vi "Auto_New.vi"() -> ()   [LabVIEW 2017]
uses:
  Control/Saurabh/prosucer_consumer_enum1.ctl
  <vilib>/Utility/error.llb/DialogType.ctl
  <vilib>/addons/database/Connection.llb/DB Tools Open Connec (String).vi
  Global/DATA LOG.vi
  Global/Global 1.vi
  <vilib>/addons/database/NI_Database_API.lvlib
panel:
  out "SHIFT":string
  in  "BARCODE RECIPE":string(combo)
  out "PLC COM.":bool
  out "SHIFT_DATA":string[](array[string])
  out "stop":bool
  out "error out 2":errorcluster
  out "Shift 4":i32
  out "Time Stamp Out":timestamp[](array[timestamp]) format="%<%X>T"
  out "Time Stamp Out 4":timestamp[](array[timestamp]) format="%<%X>T"
  out "Shift_change":bool
  out "appended array":string[][](array[string])
  out "SHIFT_DATA 2":string[](array[string])
  in  "error in (no error)":errorcluster
  in  "Tab Control":enum32{"Screen 1", "Screen 2"}(tab)
  out "OP 50":bool
  out "OP 40":bool
  out "OP 30":bool
  out "OP - 50":T1 {"RH Motor Screw" format="%#_g N-m"; "LH Motor Screw" format="%#_g N-m"; "Nut Torque" format="%#_g N-m"}
  out "OP - 40":T2 {"Stack Load" format="%#_g kg"; "Dispalcement" format="%#.3g mm"; "LH Screw" format="%#_g N-m"; "RH Screw" format="%#_g N-m"}
  out "OP - 30":T3 {"Shaft Press Load" format="%#_g kg"; "Displacement" format="%#_g mm"}
  in  "stop 2":bool
  out "OP - 10":T4 {"Leak Rate" format="%#_g sccm"}
  in  "SIMULATE INPUT":bool[](array[boolean])=[FALSE, FALSE, FALSE, FALSE]
  out "OP - 20":T5 {"Top Load" format="%#_g mm"; "Top Displace" format="%#_g mm"; "Bottom Load" format="%#_g kg"; "Bottom Displace" format="%#_g mm"}
  out "OP 10 & 20":bool
  out "OP - 60":T6 {"Screw 6" format="%#_g N-m"; "Screw 5" format="%#_g N-m"; "Screw 4" format="%#_g N-m"; "Screw 3" format="%#_g N-m"; "Screw 2" format="%#_g N-m"; "Screw 1" format="%#_g N-m"}
  out "OP - 70":T7 {"Full Open" format="%#_g V"; "Full Close" format="%#_g V"}
  out "OP - 110":cluster{"BARCODE":string}
  out "OP - 80":T8 {"Plug Press Load" format="%#_g kg"}
  out "OP - 90":T9 {"Steam Leak" format="%#_g sccm"; "Seat Leak" format="%#_g LPM"}
  out "OP - 100":T10 {"Response Time REV" format="%#_g msec"; "Response time FWD" format="%#_g msec"; "Motor Full Open" format="%#_g V"; "Motor Start Back" format="%#_g V"; "Motor Full Close" format="%#_g V"; "Motor Start Of Close" format="%#_g V"; "Motor Peak" format="%#_g A"; "Sensor O/P Full Close" format="%#_g V"; "Sensor O/P Start Of Close" format="%#_g V"; "Sensor O/P Open" format="%#_g V"}
  out "OP 60":bool
  out "OP 70 & 80":bool
  out "OP 90 -100 - 110":bool
  # "Op10 20\nOp30\nOp 40\nOp50\nOp60\nOp70-80\nOp 90-100-110"
  # "SENSOR MIN VLTG"
  # "OP - 50"
  # "OP - 40"
  # "OP - 30"
  # "OP - 10"
  # "OP - 20"
  # "OP - 60"
  # "OP - 70"
  # "OP - 110"
  # "OP - 80"
  # "OP - 90"
  # "OP - 100"
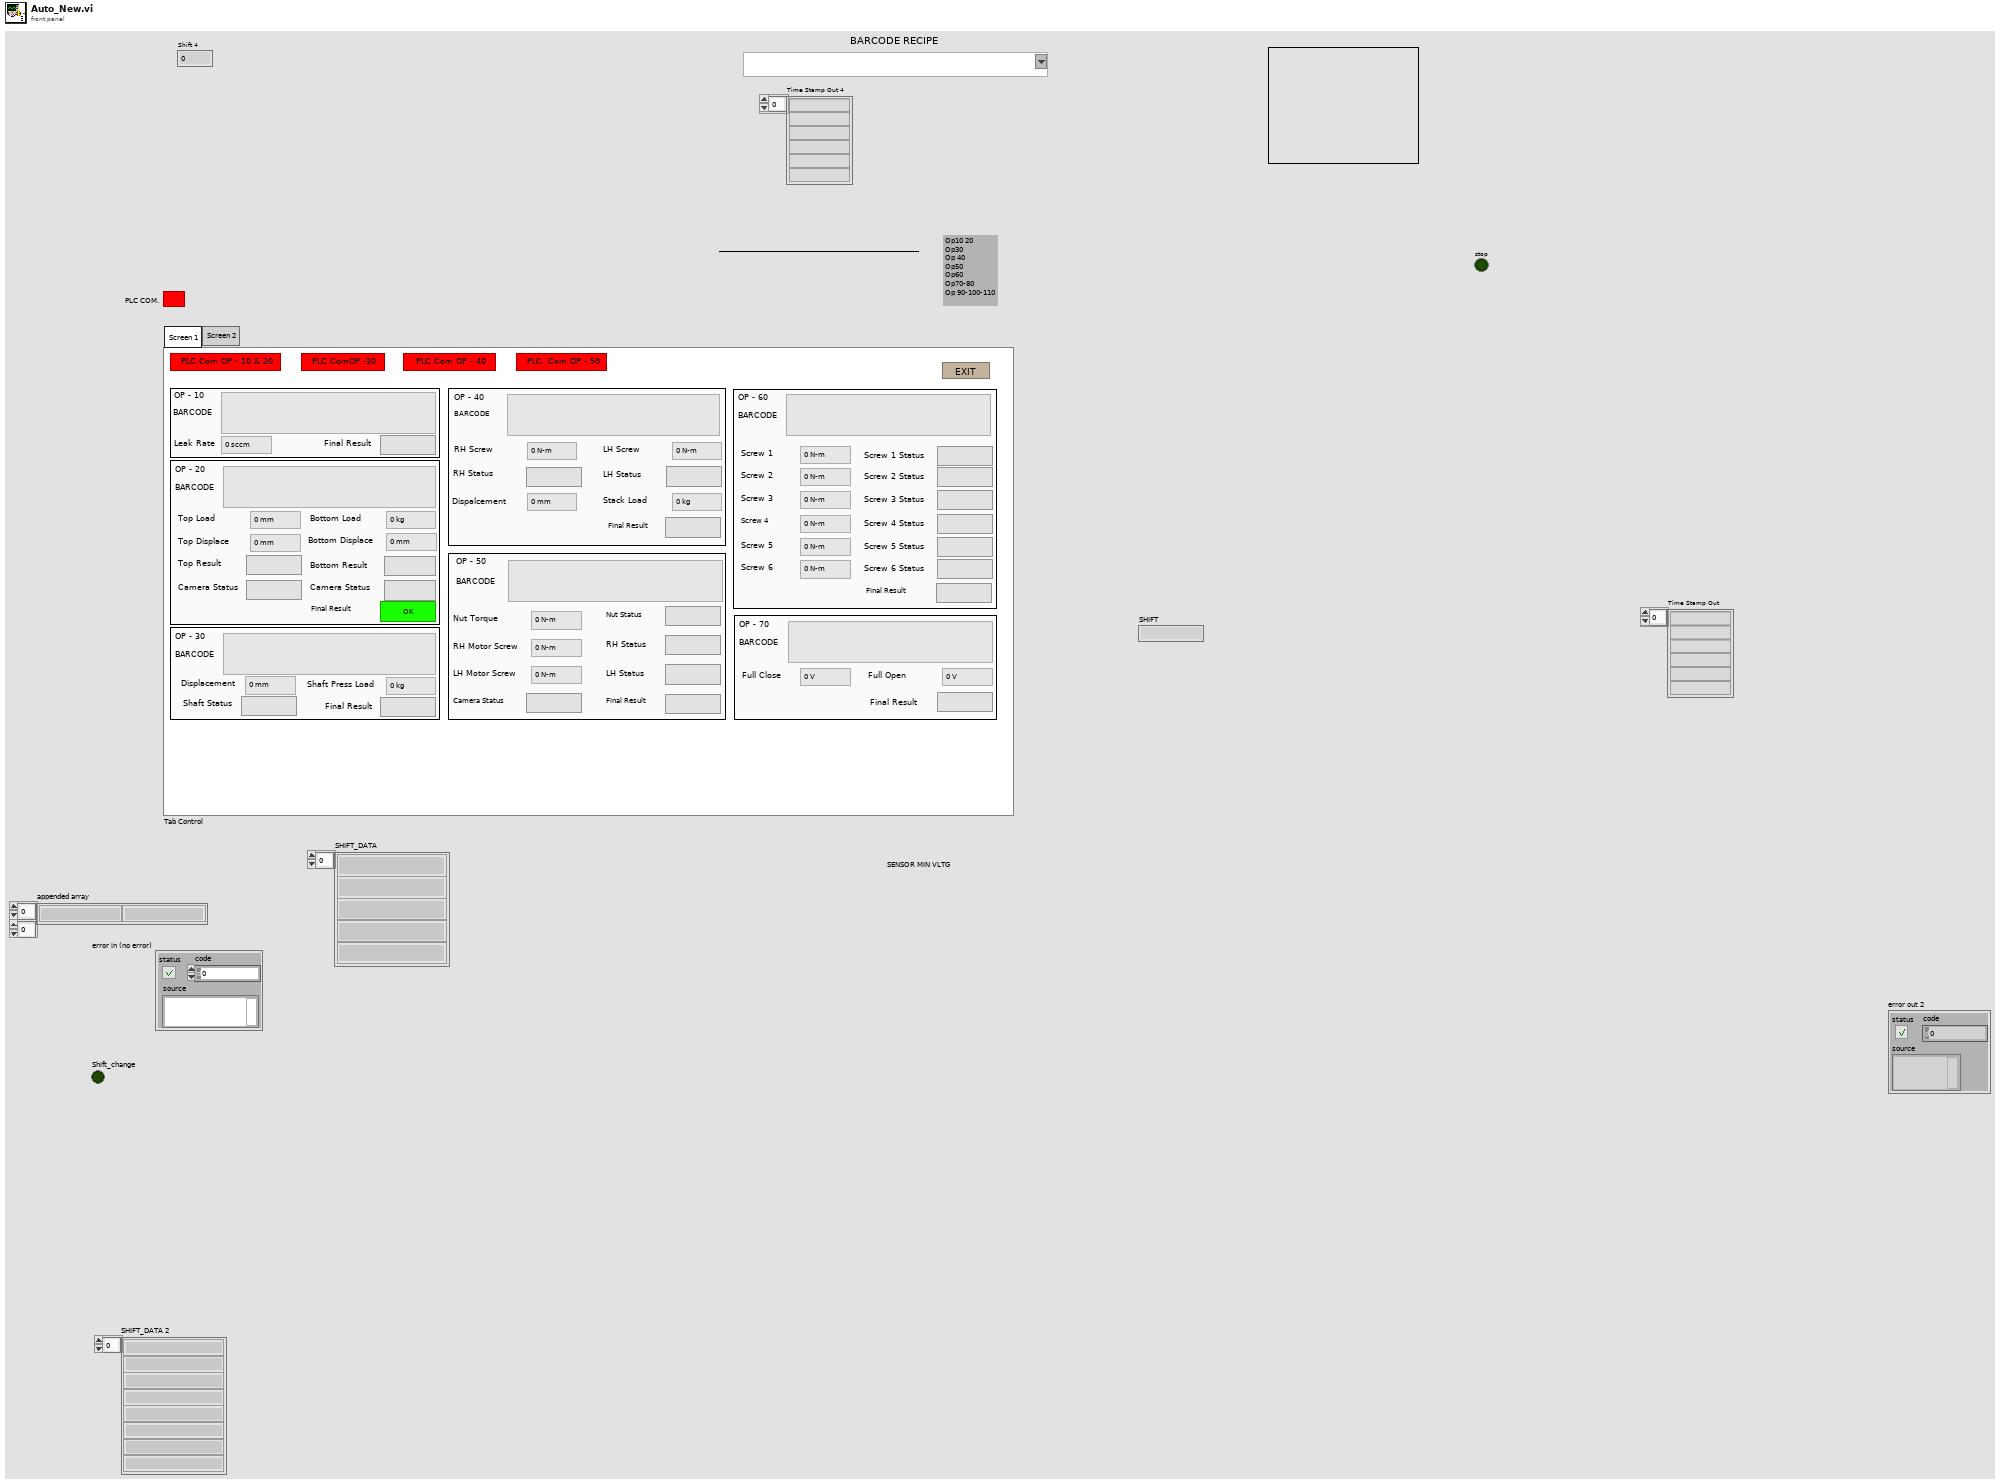
[diagram p1: front panel]
types:
  T1 = cluster{"BARCODE":string, "Nut Torque":dbl, "LH Motor Screw":dbl, "LH Status":bool, "RH Status":bool, "RH Motor Screw":dbl, "Final Result":bool, "Nut Status":bool, "Camera Status":bool}
  T2 = cluster{"BARCODE":string, "RH Screw":dbl, "LH Screw ":dbl, "RH Status":bool, "LH Status":bool, "Dispalcement ":dbl, "Stack Load ":dbl, "Final Result":bool}
  T3 = cluster{"BARCODE":string, "Displacement":dbl, "Shaft Press Load":dbl, "Shaft Status":bool, "Final Result":bool}
  T4 = cluster{"BARCODE":string, "Leak Rate":dbl, "Final Result":bool}
  T5 = cluster{"BARCODE":string, "Bottom Displace":dbl, "Bottom Load":dbl, "Camera Status":bool, "Bottom Result":bool, "Top Displace":dbl, "Top Load ":dbl, "Camera Status":bool, "Top Result":bool, "Final Result":bool}
  T6 = cluster{"BARCODE":string, "Screw 1":dbl, "Screw 2":dbl, "Screw 1 Status":bool, "Screw 2 Status":bool, "Screw 3":dbl, "Final Result":bool, "Screw 3 Status":bool, "Screw 4":dbl, "Screw 5":dbl, "Screw 4 Status":bool, "Screw 5 Status":bool, "Screw 6":dbl, "Screw 6 Status":bool}
  T7 = cluster{"BARCODE":string, "Full Close":dbl, "Full Open":dbl, "Final Result":bool}
  T8 = cluster{"BARCODE":string, "Plug Press Load":dbl, "Final Result":bool, "Loctite Status":bool}
  T9 = cluster{"BARCODE":string, "Seat Leak":dbl, "Seat Status":bool, "Steam Leak":dbl, "Final Result":bool}
  T10 = cluster{"BARCODE":string, "Sensor O/P Open":dbl, "Sensor O/P Start Of Close":dbl, "Final Result":bool, "Sensor O/P Full Close":dbl, "Motor Peak":dbl, "Motor Start Of Close":dbl, "Motor Full Close":dbl, "Motor Start Back":dbl, "Motor Full Open":dbl, "Response time FWD":dbl, "Response Time REV":dbl}
  T11 = cluster{"OP - 10":cluster{"BARCODE":string, "LEAK RATE":dbl, "RESULT":bool}, "OP - 30":cluster{"BARCODE":string, "Displacement":dbl, "Load":dbl, "Middle Gear Shaft Status":bool, "Final Result":bool}, "OP - 60":cluster{"BARCODE":string, "Screw 1 Data":dbl, "Screw 2 data":dbl, "Screw 1 Status":bool, "Screw 2 Status":bool, "Screw3 Data":dbl, "Final Result":bool, "Screw3 Status":bool, "Screw4 Data":dbl, "Screw5 Data":dbl, "Screw4 Status":bool, "Screw5 Status":bool, "Screw6 Data":dbl, "Screw6 Status":bool}, "OP - 70":cluster{"BARCODE":string, "Sensor MIN Vltg":dbl, "Sensor MAX Vltg":dbl, "Final Result":bool}, "OP - 80":cluster{"BARCODE":string, "Load":dbl, "Final Result":bool, "Dispensing":bool}, "OP - 90":cluster{"BARCODE":string, "Seat LT Data":dbl, "Seat Status":bool, "Steam LT Data":dbl, "Final Result":bool}, "OP - 100":cluster{"BARCODE":string, "Sensor O/P Open V":dbl, "Start Of Close Sensor V":dbl, "Final Result":bool, "Sensor O/P Full Close V":dbl, "Response Time FWD (mSec)":dbl, "Response Time REV (mSec)":dbl, "Motor V Start Of Close A":dbl, "Motor V Full Close B R":dbl, "Motor V Start Back C":dbl, "Motor V Full Open D":dbl, "Motor RMS Current A":dbl}, "OP - 110":cluster{"BARCODE":string}, "OP - 20":cluster{"BARCODE":string, "Bottom Displace":dbl, "Bottom Load":dbl, "Camera Status":bool, "Bottom Result":bool, "Top Displace":dbl, "Top Load ":dbl, "Camera Status":bool, "Top Result":bool, "Final Result":bool}, "OP - 40":cluster{"BARCODE":string, "RH Screw":dbl, "LH Screw ":dbl, "RH Status":bool, "LH Status":bool, "Dispalcement ":dbl, "Stack Load ":dbl, "Final Result":bool}, "OP - 50":cluster{"BARCODE":string, "Nut Torque":dbl, "LH Motor Screw":dbl, "LH Status":bool, "RH Status":bool, "RH Motor Screw":dbl, "Final Result":bool, "Nut Status":bool, "Camera Status":bool}}
  T12 = typedef "prosucer_consumer_enum1.ctl" = enum16{"-1", "SCAN1", "SCAN2", "SCAN3", "SCAN4", "SCAN5", "SCAN6", "SCAN7", "SCAN8", "SCAN9", "SCAN10", "SCAN11", "STOP", "DATALOG1", "DATALOG2", "DATALOG3", "DATALOG4", "DATALOG5", "DATALOG6", "DATALOG7", "DATALOG8", "DATALOG9", "DATALOG10", "DATALOG11", "CYCLE_START1", "CYCLE_START2", "CYCLE_START3", "CYCLE_START4", "BARCODE RECIPE", "EMERGENCY STOP"}
  T13 = typedef "NI_Database_API.lvlib/Conn ObjectReference.ctl" = refnum<k1>
  T14 = typedef "DialogType.ctl" = u16
  T15 = cluster{"trimmed string":string, "SHIFT":string, "date/time string":string, string, "Input 2":string}
  T16 = cluster{"SHIFT":string, "date/time string":string, "Input 2":string, string}
  T17 = cluster{"date/time string":string, "Input 2":string, "Input 2":string, "Input 2":string, "Input 2":string, "Input 2":string, "Input 2":string, "Input 2":string, "Input 2":string, "Input 2":string, "Input 2":string}
  T18 = cluster{"date/time string":string, "SHIFT":string, "Input 2":string, "Input 2":string, "Input 2":string, "Input 2":string, "Input 2":string, "Input 2":string, "Input 2":string, "Input 2":string, "Input 2":string, "Input 2":string}
  T19 = cluster{"date/time string":string, "Input 2":string, "Input 2":string, "Input 2":string, "Input 2":string}
  T20 = cluster{"date/time string":string, "SHIFT":string, "Input 2":string, "Input 2":string, "Input 2":string, "Input 2":string}
  T21 = cluster{"date/time string":string, "Input 2":string, "Input 2":string, "Input 2":string, "Input 2":string, "Input 2":string, "Input 2":string, "Input 2":string, "Input 2":string}
  T22 = cluster{"date/time string":string, "SHIFT":string, "Input 2":string, "Input 2":string, "Input 2":string, "Input 2":string, "Input 2":string, "Input 2":string, "Input 2":string, "Input 2":string}
  T23 = cluster{"date/time string":string, "Input 2":string, "Input 2":string, "Input 2":string, "Input 2":string, "Input 2":string, "Input 2":string, "Input 2":string}
  T24 = cluster{"date/time string":string, "SHIFT":string, "Input 2":string, "Input 2":string, "Input 2":string, "Input 2":string, "Input 2":string, "Input 2":string}
  T25 = cluster{"date/time string":string, "Input 2":string, "Input 2":string, "Input 2":string, "Input 2":string, "Input 2":string, "Input 2":string, "Input 2":string, "Input 2":string, "Input 2":string, "Input 2":string, "Input 2":string, "Input 2":string}
  T26 = cluster{"date/time string":string, "SHIFT":string, "Input 2":string, "Input 2":string, "Input 2":string, "Input 2":string, "Input 2":string, "Input 2":string, "Input 2":string, "Input 2":string, "Input 2":string, "Input 2":string, "Input 2":string, "Input 2":string}
  T27 = cluster{"date/time string":string, "Input 2":string, "Input 2":string, "Input 2":string}
  T28 = cluster{"date/time string":string, "SHIFT":string, "Input 2":string, "Input 2":string, "Input 2":string}
  T29 = cluster{"BARCODE":string, "Seat LT Data":dbl, "Seat Status":bool, "Steam LT Data":dbl, "Final Result":bool}
  T30 = cluster{"BARCODE":string, "Sensor O/P Open V":dbl, "Start Of Close Sensor V":dbl, "Final Result":bool, "Sensor O/P Full Close V":dbl, "Response Time FWD (mSec)":dbl, "Response Time REV (mSec)":dbl, "Motor V Start Of Close A":dbl, "Motor V Full Close B R":dbl, "Motor V Start Back C":dbl, "Motor V Full Open D":dbl, "Motor RMS Current A":dbl}
  T31 = cluster{"BARCODE":string, "LEAK RATE":dbl, "RESULT":bool}
  T32 = cluster{"BARCODE":string, "Displacement":dbl, "Load":dbl, "Middle Gear Shaft Status":bool, "Final Result":bool}
  T33 = cluster{"BARCODE":string, "Screw 1 Data":dbl, "Screw 2 data":dbl, "Screw 1 Status":bool, "Screw 2 Status":bool, "Screw3 Data":dbl, "Final Result":bool, "Screw3 Status":bool, "Screw4 Data":dbl, "Screw5 Data":dbl, "Screw4 Status":bool, "Screw5 Status":bool, "Screw6 Data":dbl, "Screw6 Status":bool}
  T34 = cluster{"BARCODE":string, "Sensor MIN Vltg":dbl, "Sensor MAX Vltg":dbl, "Final Result":bool}
  T35 = cluster{"BARCODE":string, "Load":dbl, "Final Result":bool, "Dispensing":bool}
  T36 = enum32{"invalid app kind", "Development System", "Run Time System", "Student Edition", "Embedded LabVIEW", "Evaluation", "Custom"}
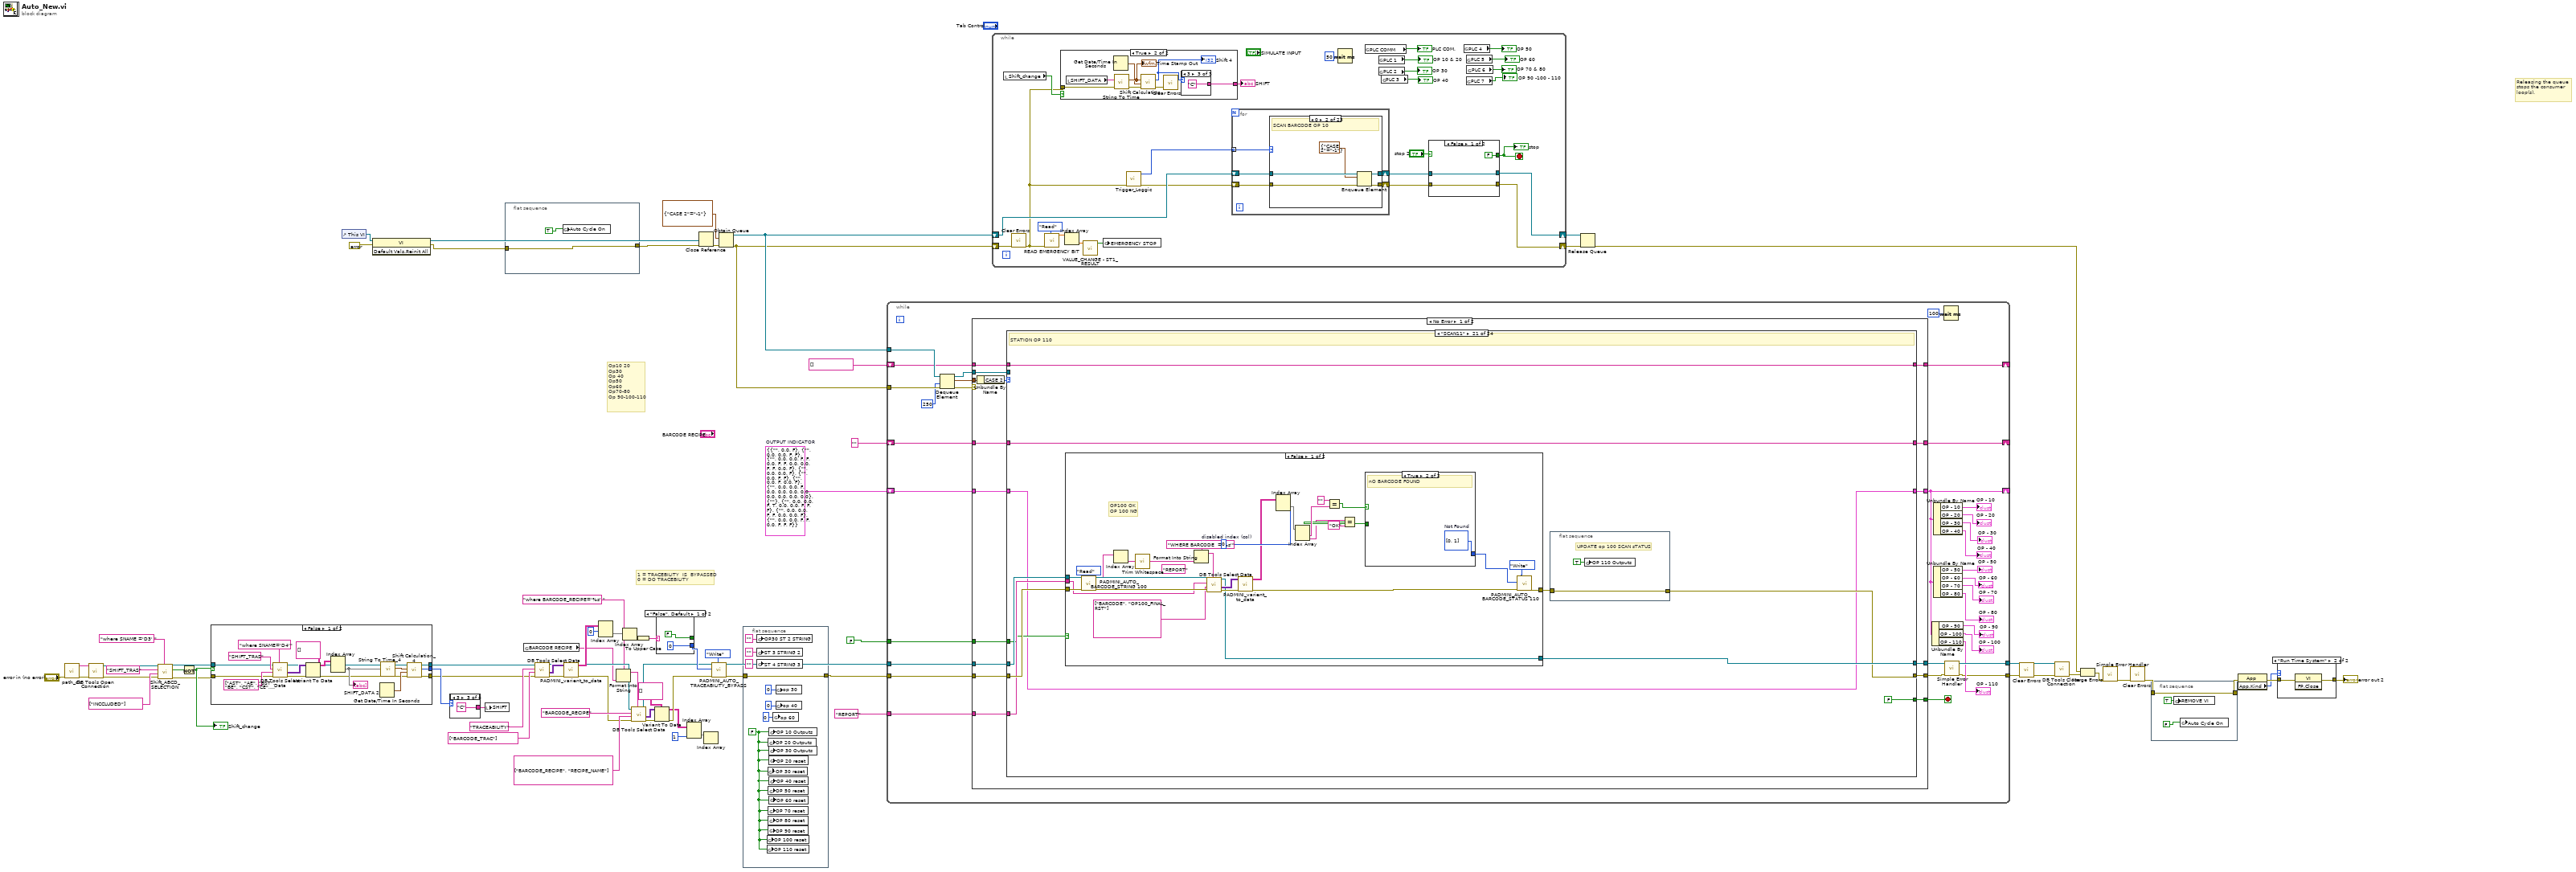
[diagram p0: block diagram]
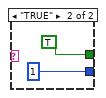
[diagram p2: hidden frame]
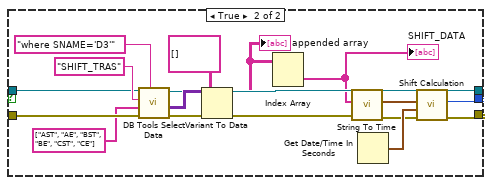
[diagram p3: hidden frame]
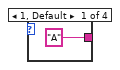
[diagram p4: hidden frame]
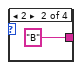
[diagram p5: hidden frame]
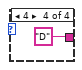
[diagram p6: hidden frame]
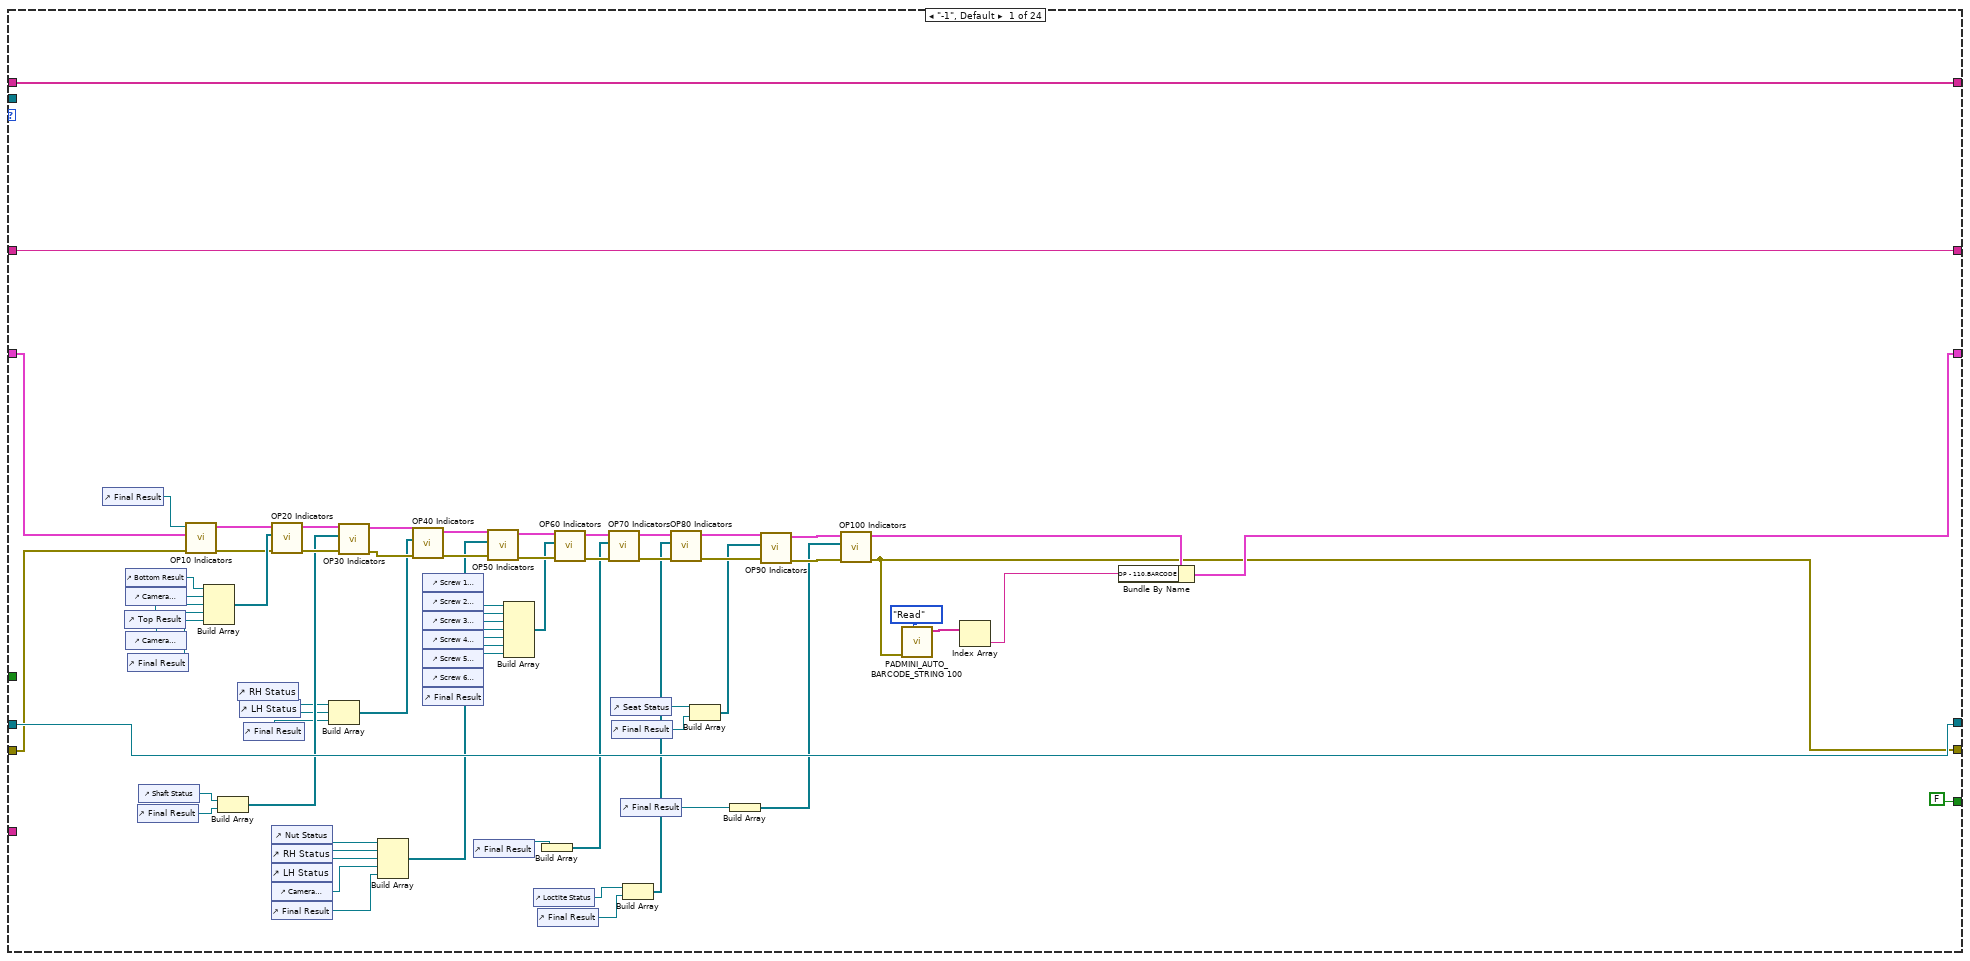
[diagram p7: hidden frame]
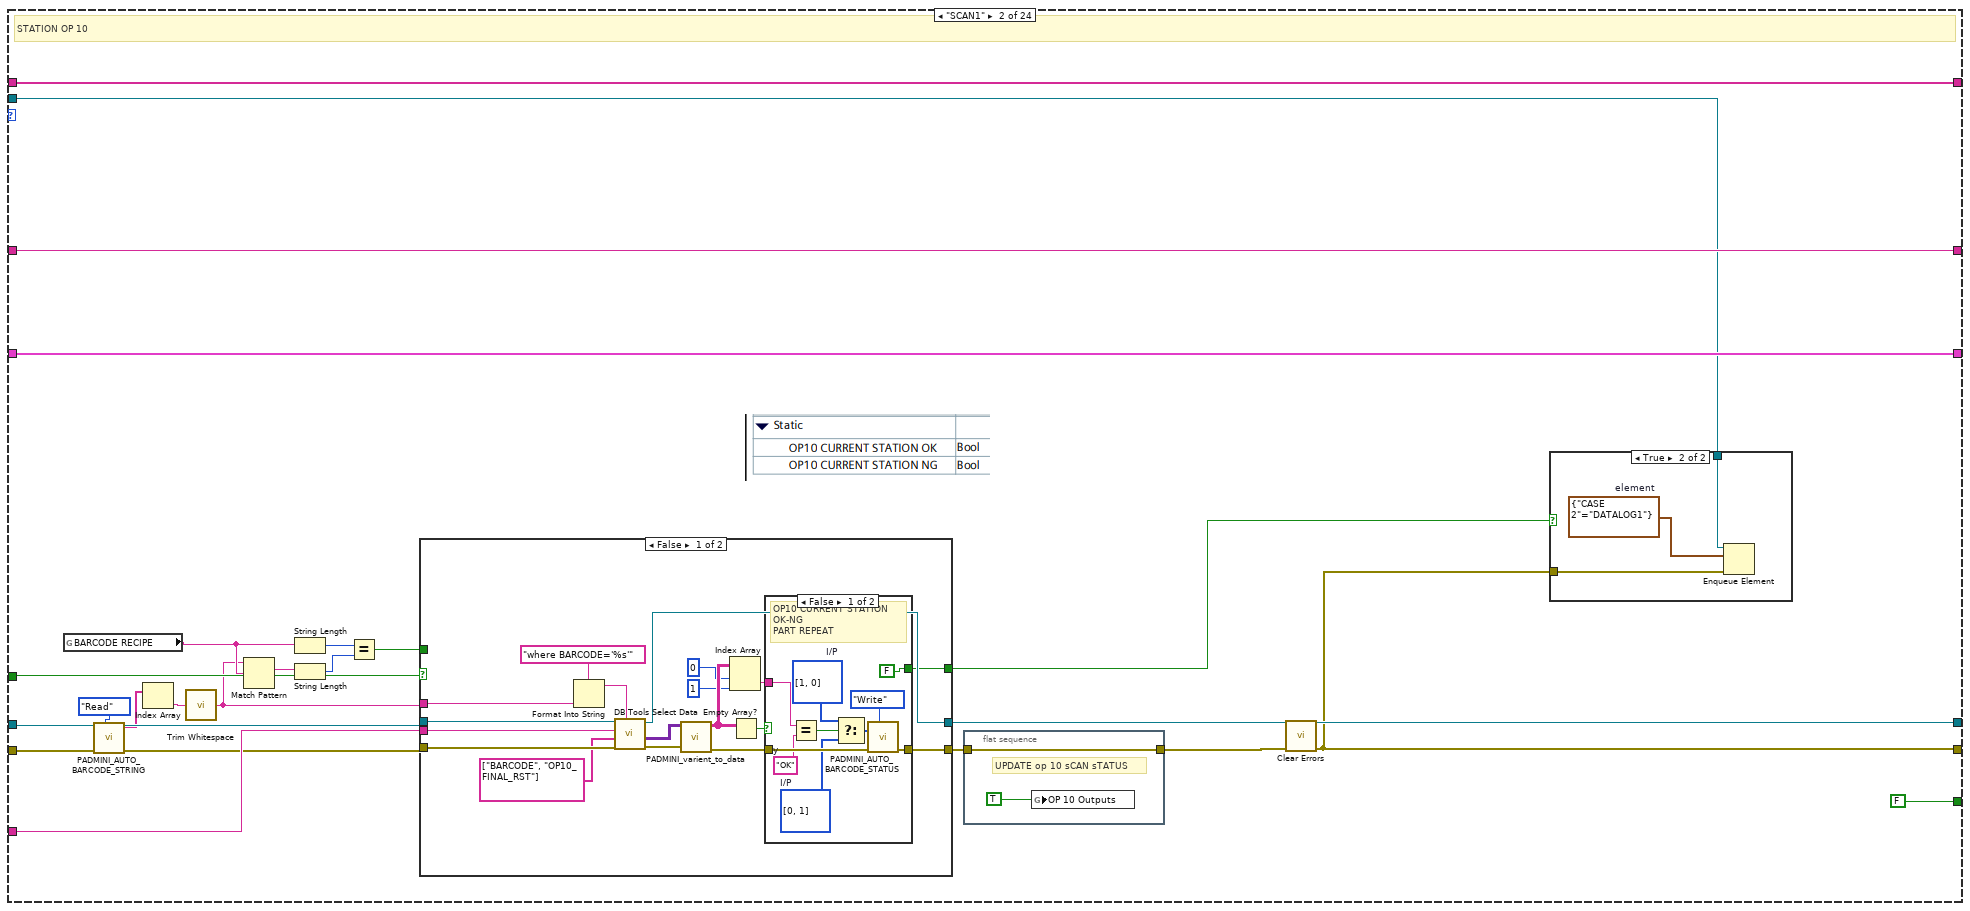
[diagram p8: hidden frame]
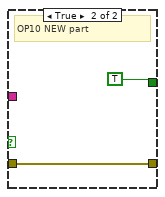
[diagram p10: hidden frame]
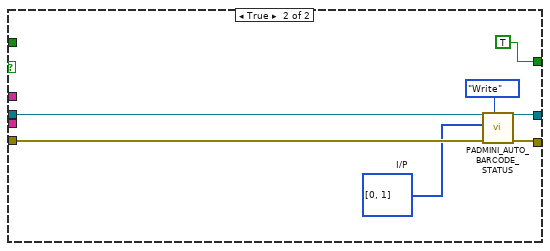
[diagram p11: hidden frame]
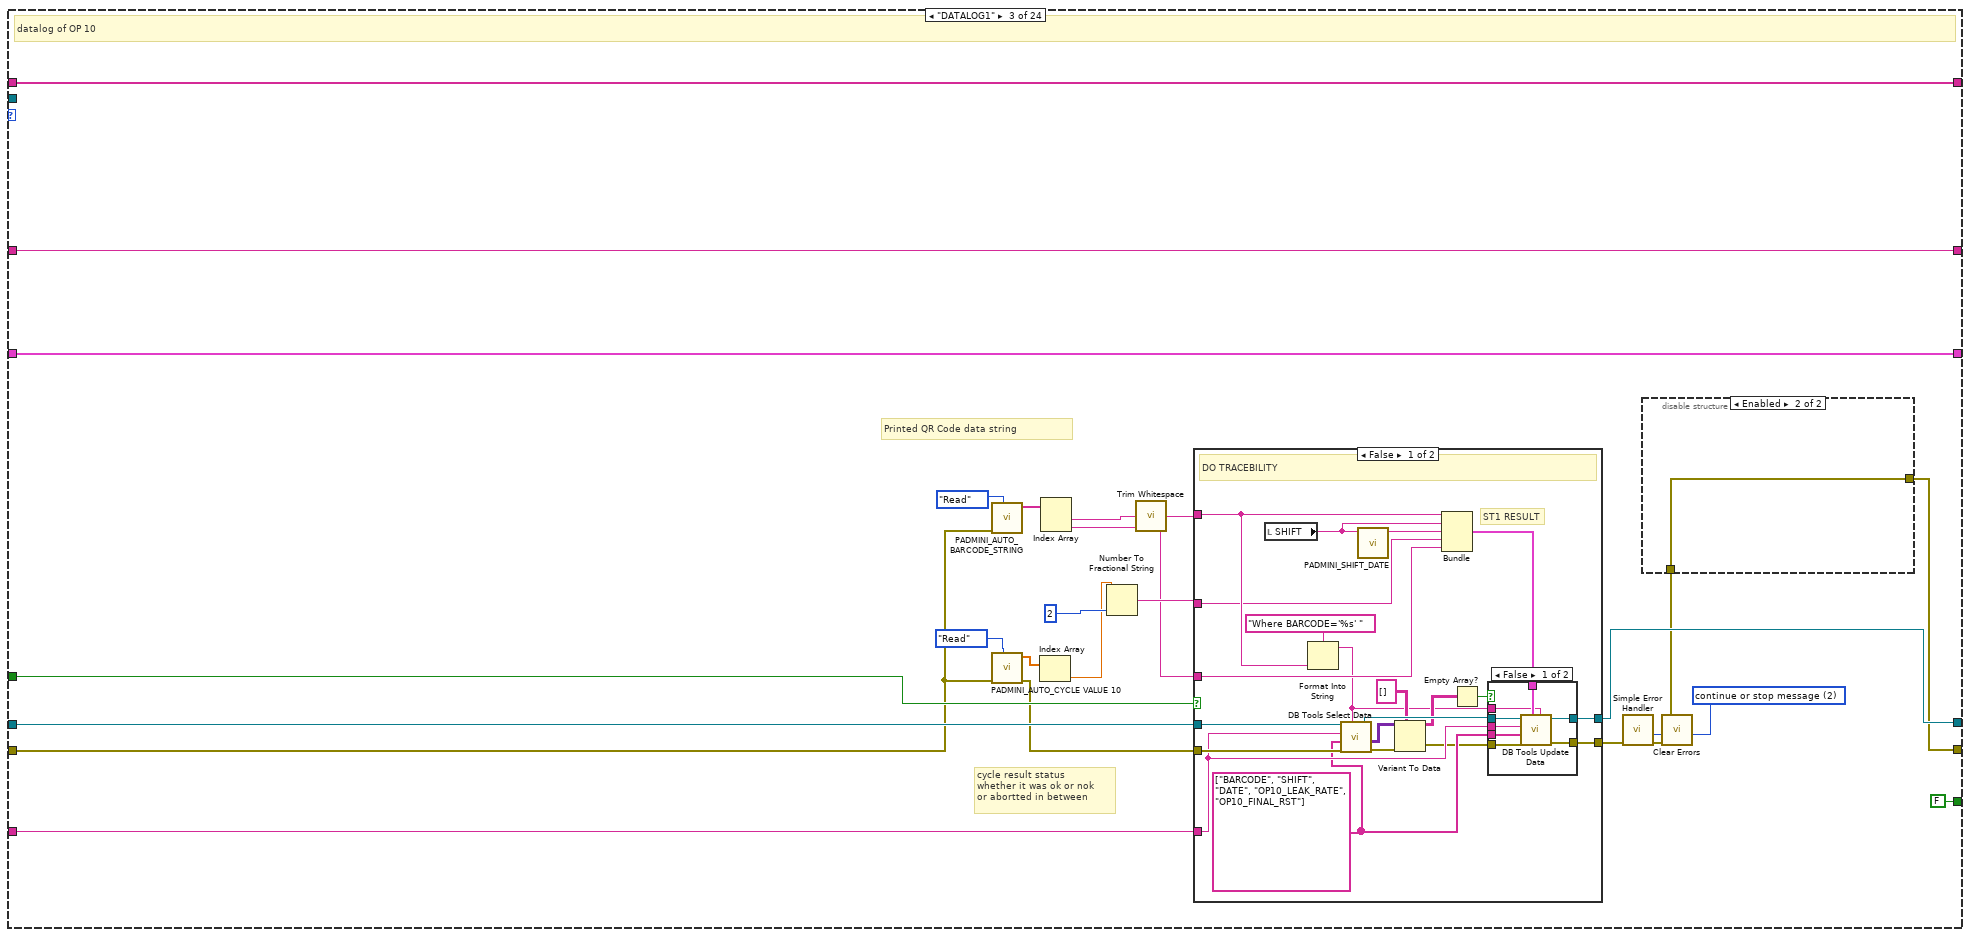
[diagram p12: hidden frame]
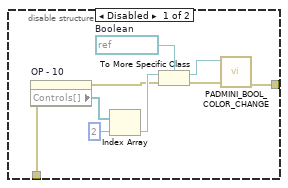
[diagram p13: hidden frame]
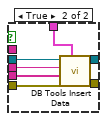
[diagram p14: hidden frame]
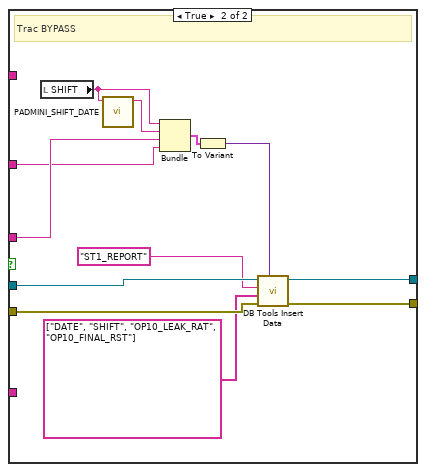
[diagram p15: hidden frame]
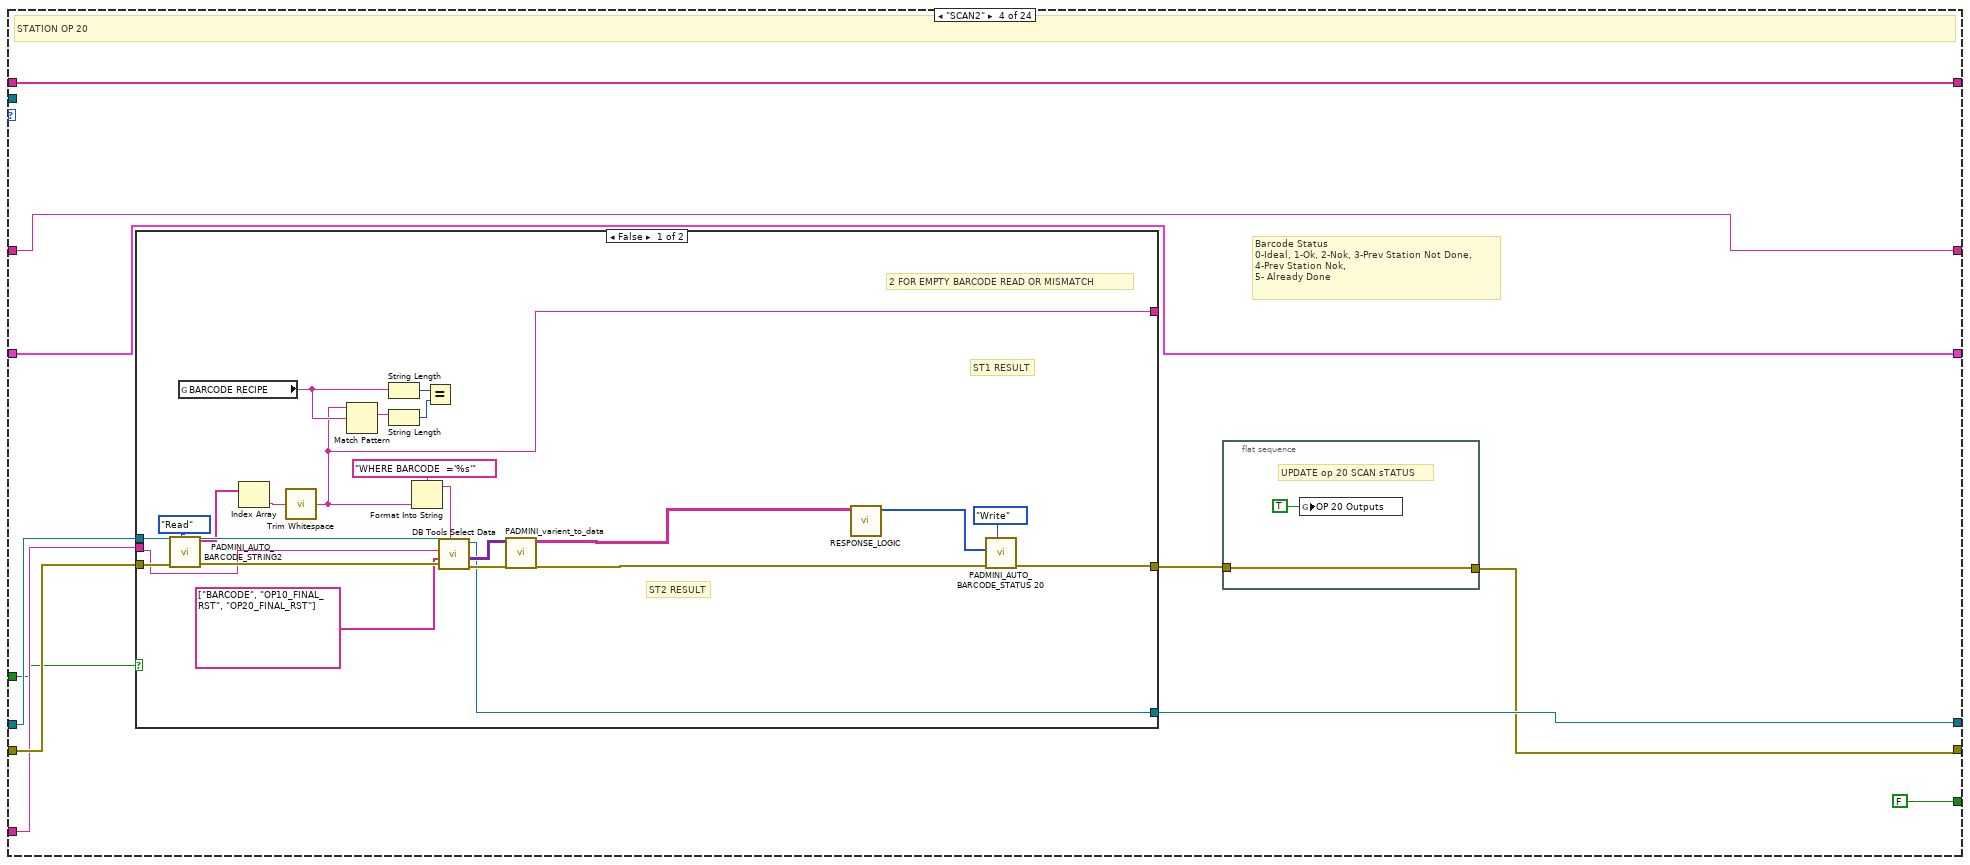
[diagram p16: hidden frame]
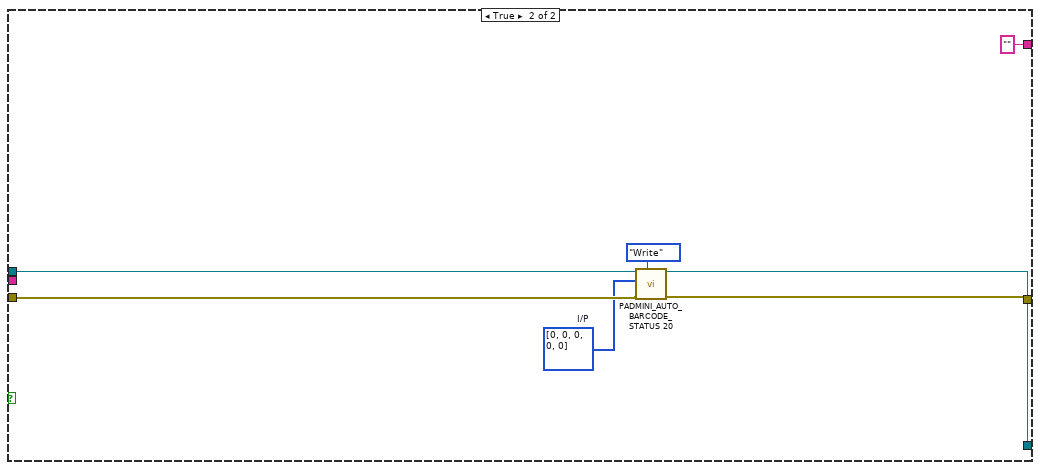
[diagram p17: hidden frame]
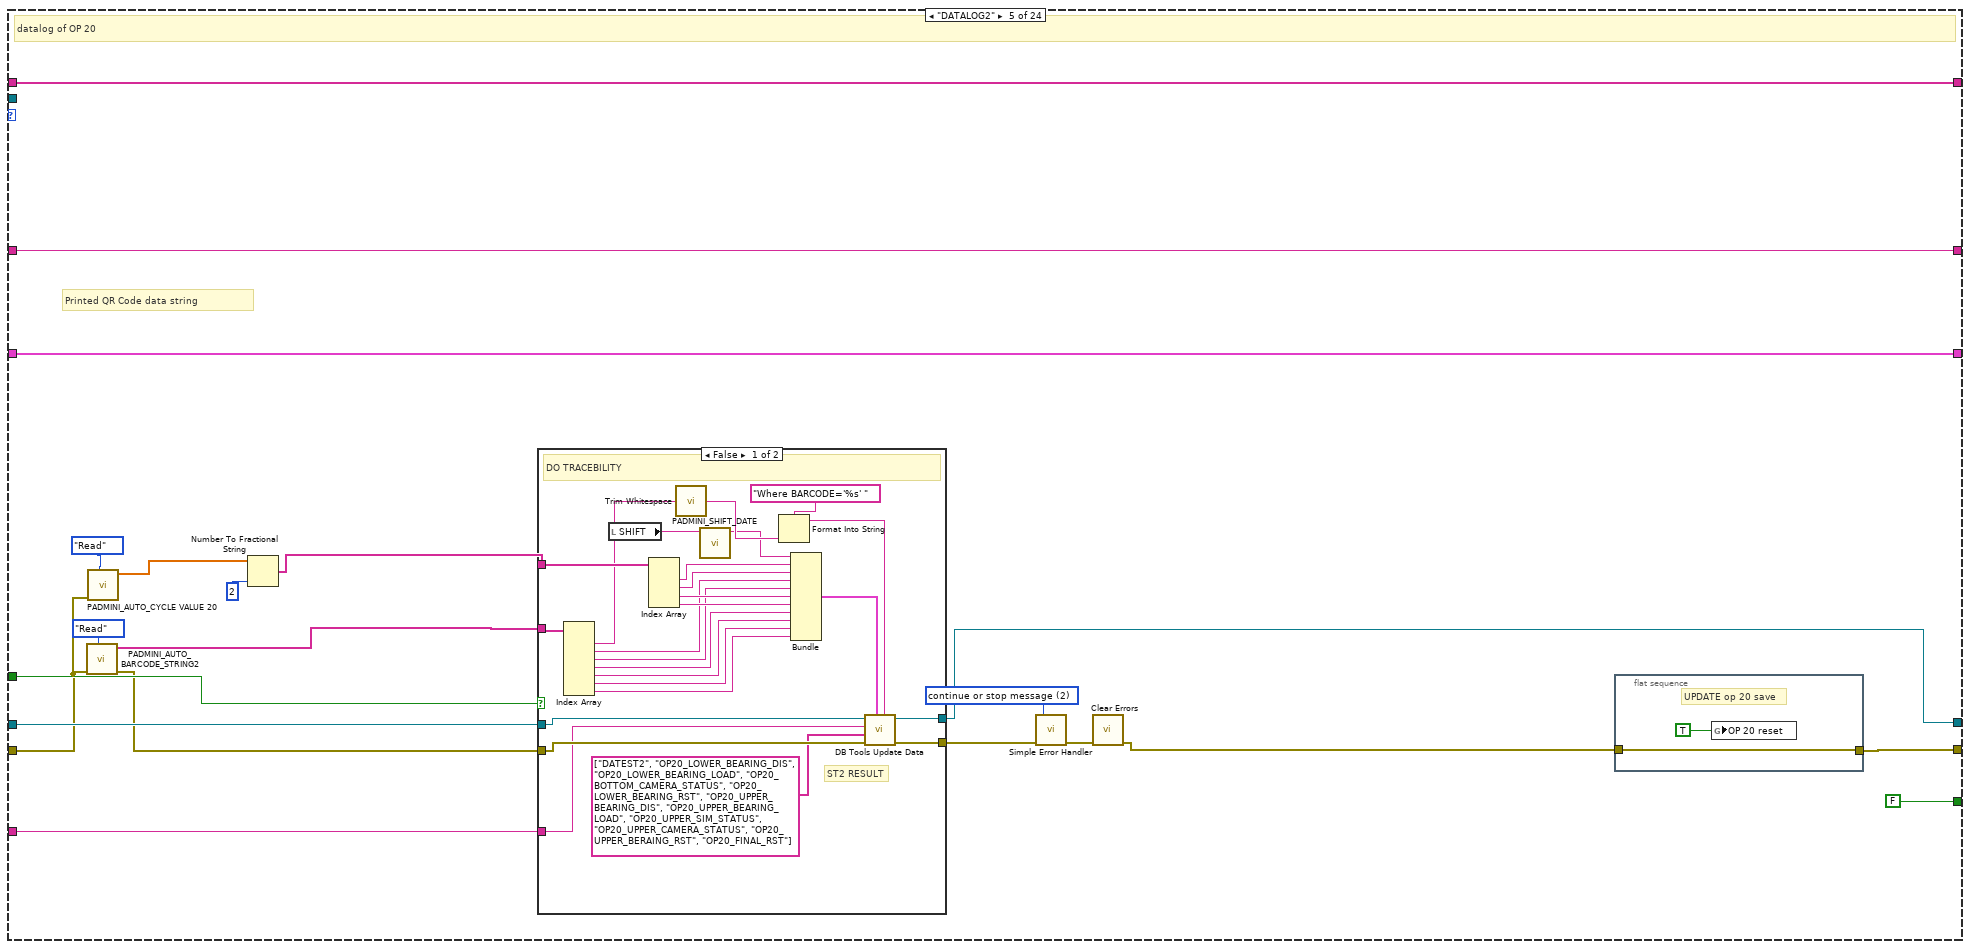
[diagram p18: hidden frame]
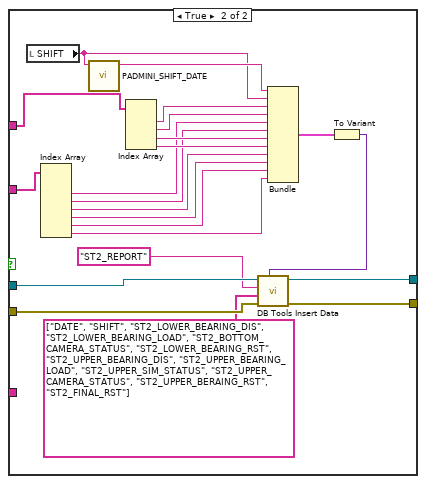
[diagram p19: hidden frame]
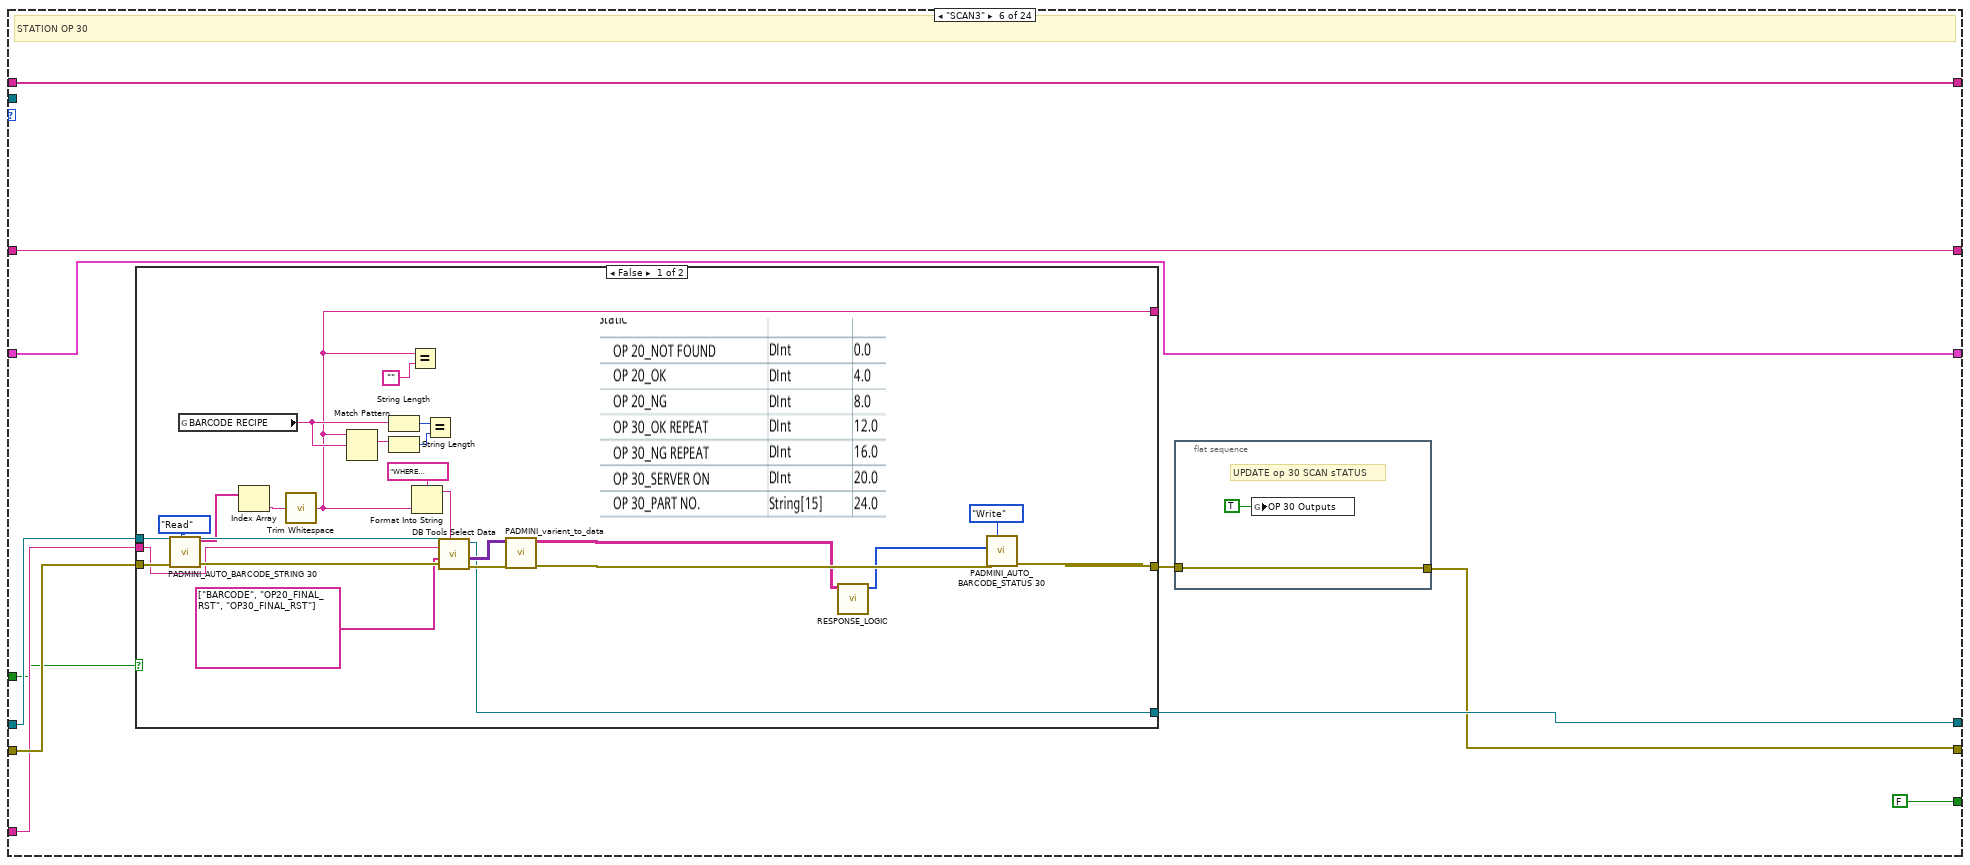
[diagram p20: hidden frame]
diagram:
  w3 = T11 {"OP - 10"={"BARCODE"="", "LEAK RATE"=0.0, "RESULT"=FALSE}, "OP - 30"={"BARCODE"="", "Displacement"=0.0, "Load"=0.0, "Middle Gear Shaft Status"=FALSE, "Final Result"=FALSE}, "OP - 60"={"BARCODE"="", "Screw 1 Data"=0.0, "Screw 2 data"=0.0, "Screw 1 Status"=FALSE, "Screw 2 Status"=FALSE, "Screw3 Data"=0.0, "Final Result"=FALSE, "Screw3 Status"=FALSE, "Screw4 Data"=0.0, "Screw5 Data"=0.0, "Screw4 Status"=FALSE, "Screw5 Status"=FALSE, "Screw6 Data"=0.0, "Screw6 Status"=FALSE}, "OP - 70"={"BARCODE"="", "Sensor MIN Vltg"=0.0, "Sensor MAX Vltg"=0.0, "Final Result"=FALSE}, "OP - 80"={"BARCODE"="", "Load"=0.0, "Final Result"=FALSE, "Dispensing"=FALSE}, "OP - 90"={"BARCODE"="", "Seat LT Data"=0.0, "Seat Status"=FALSE, "Steam LT Data"=0.0, "Final Result"=FALSE}, "OP - 100"={"BARCODE"="", "Sensor O/P Open V"=0.0, "Start Of Close Sensor V"=0.0, "Final Result"=FALSE, "Sensor O/P Full Close V"=0.0, "Response Time FWD (mSec)"=0.0, "Response Time REV (mSec)"=0.0, "Motor V Start Of Close A"=0.0, "Motor V Full Close B R"=0.0, "Motor V Start Back C"=0.0, "Motor V Full Open D"=0.0, "Motor RMS Current A"=0.0}, "OP - 110"={"BARCODE"=""}, "OP - 20"={"BARCODE"="", "Bottom Displace"=0.0, "Bottom Load"=0.0, "Camera Status"=FALSE, "Bottom Result"=TRUE, "Top Displace"=0.0, "Top Load "=0.0, "Camera Status"=FALSE, "Top Result"=FALSE, "Final Result"=FALSE}, "OP - 40"={"BARCODE"="", "RH Screw"=0.0, "LH Screw "=0.0, "RH Status"=FALSE, "LH Status"=FALSE, "Dispalcement "=0.0, "Stack Load "=0.0, "Final Result"=FALSE}, "OP - 50"={"BARCODE"="", "Nut Torque"=0.0, "LH Motor Screw"=0.0, "LH Status"=FALSE, "RH Status"=FALSE, "RH Motor Screw"=0.0, "Final Result"=FALSE, "Nut Status"=FALSE, "Camera Status"=FALSE}}  # OUTPUT INDICATOR
  # "Op10 20\nOp30\nOp 40\nOp50\nOp60\nOp70-80\nOp 90-100-110"
  # "1 = TRACEBILITY  IS  BYPASSED\n0 = DO TRACEBILITY"
  # "Releasing the queue stops the consumer loop(s)."
  n1 = call "path_db.vi"("error in"="error in (no error)") -> ("error out"=w48:errorcluster, "resulting string"=w69:string)  [unwired: 9 in]
  n2 = call-poly <vilib>:"DB Tools Open Connection.vi"("error in (no error)"=w48, "connection information"=w69) -> ("error out"=w47:errorcluster, "connection reference"=w41:T13)  [unwired: 6 in]
  n3 = call "Shift_ABCD_SELECTION.vi"("Where"="where SNAME ='D3' ", "error in (no error)"=w47, "Array"=string[] ["INCCLUDED"], "table"="SHIFT_TRAS", "Refnum in"=w41) -> ("error out"=w5:errorcluster, "Boolean"=w60:bool, "Refnum out"=w61:T13)  [unwired: 4 in]
  n4 = Not(x=w60) -> (.not. x?=w59:bool)
  "Shift_change" <- w59
  n5 = case shown="False" w59 {
    tunnel: [w74 w98] -> w65
    tunnel: w61 -> [w77 w96]
    tunnel: w5 -> [w76 w95]
    tunnel: [w75 w94] -> w30
    tunnel: [w73 w88] -> w29
    frame False {
      n6 = call <vilib>:"DB Tools Select Data.vi"("condition"="where SNAME='D4'", "error in (no error)"=w76, "columns"=string[] ["AST", "AE", "BST", "BE", "CST", "CE", "DST", "DE"], "table"="SHIFT_TRAS", "connection reference"=w77) -> ("error out"=w83:errorcluster, "data"=w87:variant[][], "connection reference out"=w75:T13)  [unwired: 1 in]
      n7 = Variant To Data(error in=w83, type=string[][] [], Variant=w87) -> (data=w80:string[][], error out=w73:errorcluster)
      n8 = Index Array(array=w80) -> (element=w79:string[])  [unwired: 2 in]
      "SHIFT_DATA 2" <- w79
      n9 = Get Date/Time In Seconds() -> (seconds since 1Jan1904=w82:timestamp)
      n10 = call "String To Time_4.vi"("String Array In"=w79) -> ("Time Stamp Out"=w78:timestamp[])  [unwired: 9 in, 1 out]
      n11 = call "Shift Calculation_4.vi"("Current Time"=w82, "Time Stamp Out"=w78) -> ("Shift"=w74:i32)  [unwired: 8 in, 1 out]
    }
    frame True {
      n12 = call <vilib>:"DB Tools Select Data.vi"("condition"="where SNAME='D3'", "error in (no error)"=w95, "columns"=string[] ["AST", "AE", "BST", "BE", "CST", "CE"], "table"="SHIFT_TRAS", "connection reference"=w96) -> ("error out"=w100:errorcluster, "data"=w104:variant[][], "connection reference out"=w94:T13)  [unwired: 1 in]
      n13 = Variant To Data(error in=w100, type=string[][] [], Variant=w104) -> (data=w92:string[][], error out=w90:errorcluster)
      "appended array" <- w92
      n14 = Index Array(array=w92) -> (element=w91:string[])  [unwired: 2 in]
      "SHIFT_DATA" <- w91
      n15 = call "String To Time.vi"("error in (no error)"=w90, "String Array In"=w91) -> ("error out"=w89:errorcluster, "Time Stamp Out"=w97:timestamp[])  [unwired: 8 in]
      n16 = Get Date/Time In Seconds() -> (seconds since 1Jan1904=w99:timestamp)
      n17 = call "Shift Calculation.vi"("error in (no error)"=w89, "Current Time"=w99, "Time Stamp Out"=w97) -> ("error out"=w88:errorcluster, "Shift"=w98:i32)  [unwired: 7 in]
    }
  }
  n18 = control-ref of="This VI"() -> (w45:refnum<vi>)
  n19 = invoke class="VI" method="Default Vals.Reinit All"(reference=w45, error in=errorcluster {"status"=FALSE, "code"=0, "source"=""} ("error in (no error)")) -> (reference out=w44:refnum<vi>, error out=w1:errorcluster)  [unwired: 1 in, 1 out]
  n20 = case shown="3" w65 {
    tunnel: ["A" "B" "C" "D"] -> w58
    frame 1, Default {
    }
    frame 2 {
    }
    frame 3 {
    }
    frame 4 {
    }
  }
  n21 = local write "SHIFT"(w58) -> ()
  n22 = flat-sequence {
    tunnel: [w110] -> w2
    tunnel: w1 -> [w110]
    frame #0 {
      n23 = global write "DATA LOG.vi" "Auto Cycle On"(TRUE) -> ()
    }
  }
  n24 = global read "Global 1.vi" "BARCODE RECIPE"() -> (w11:string)
  n25 = call <vilib>:"DB Tools Select Data.vi"("error in (no error)"=w29, "columns"=string[] ["BARCODE_TRAC"], "table"="TRACEABILITY", "connection reference"=w30) -> ("error out"=w39:errorcluster, "data"=w38:variant[][], "connection reference out"=w17:T13)  [unwired: 2 in]
  n26 = call "PADMINI_varient_to_data.vi"("error in (no error)"=w39, "data"=w38) -> ("error out"=w15:errorcluster, "Array"=w37:string[][])  [unwired: 8 in]
  n27 = Index Array(array=w37, index (row)=0 ("disabled index (col)")) -> (element=w36:string[])  [unwired: 1 in]
  n28 = Format Into String(format string="where BARCODE_RECIPE='%s' ", w11) -> (resulting string=w9:string)  [unwired: 2 in, 1 out]
  n29 = Index Array(array=w36) -> (element=w32:string)  [unwired: 1 in]
  n30 = call <vilib>:"DB Tools Select Data.vi"("condition"=w9, "error in (no error)"=w15, "columns"=string[] ["BARCODE_RECIPE", "RECIPE_NAME"], "table"="BARCODE_RECIPE", "connection reference"=w17) -> ("error out"=w19:errorcluster, "data"=w18:variant[][], "connection reference out"=w16:T13)  [unwired: 1 in]
  n31 = To Upper Case(1:w32) -> (0:w31:string)
  n32 = Variant To Data(error in=w19, type=string[][] [], Variant=w18) -> (data=w12:string[][], error out=w14:errorcluster)
  n33 = case shown="\"False\", Default" w31 {
    tunnel: [FALSE ("BARCODE TRACEABILITY") TRUE ("BARCODE TRACEABILITY")] -> _
    tunnel: [0 1] -> w27
    frame "False", Default {
    }
    frame "TRUE" {
    }
  }
  n34 = Index Array(array=w12, index (col)=1 ("disabled index (col)")) -> (element=w7:string[])  [unwired: 1 in]
  n35 = Close Reference(reference=w44, error in (no error)=w2) -> (error out=w42:errorcluster)
  n36 = Index Array(array=w7) -> ()  [unwired: 1 in, 1 out]
  n37 = call "PADMINI_AUTO_TRACEABILITY_BYPASS.vi"("Enum"=enum16{"Read", "Write"}."Write", "error in (no error)"=w14, "I/P"=w27) -> ("error out"=w25:errorcluster)  [unwired: 7 in, 1 out]
  n38 = Obtain Queue(element data type=cluster{"CASE 2":T12} {"CASE 2"=enum."-1"}, error in (no error)=w42) -> (queue out=w70:refnum<queue>, error out=w22:errorcluster)  [unwired: 3 in, 1 out]
  n39 = flat-sequence {
    tunnel: w25 -> [w119]
    tunnel: [w119] -> w24
    frame #0 {
      w115 = FALSE
      n40 = global write "DATA LOG.vi" "OP30 ST 2 STRING"("" ("OP30 ST 2 STRING")) -> ()
      n41 = global write "DATA LOG.vi" "ST 3 STRING 2"("" ("ST 3 STRING 2")) -> ()
      n42 = global write "DATA LOG.vi" "ST 4 STRING 3"("" ("ST 4 STRING 3")) -> ()
      n43 = global write "DATA LOG.vi" "OP 100 reset"(w115) -> ()
      n44 = global write "DATA LOG.vi" "OP 110 reset"(w115) -> ()
      n45 = global write "DATA LOG.vi" "OP 30 reset"(w115) -> ()
      n46 = global write "DATA LOG.vi" "OP 20 Outputs"(w115) -> ()
      n47 = global write "DATA LOG.vi" "OP 50 reset"(w115) -> ()
      n48 = global write "DATA LOG.vi" "OP 70 reset"(w115) -> ()
      n49 = global write "DATA LOG.vi" "OP 80 reset"(w115) -> ()
      n50 = global write "DATA LOG.vi" "OP 90 reset"(w115) -> ()
      n51 = global write "DATA LOG.vi" "OP 10 Outputs"(w115) -> ()
      n52 = global write "DATA LOG.vi" "OP 30 Outputs"(w115) -> ()
      n53 = global write "DATA LOG.vi" "OP 20 reset"(w115) -> ()
      n54 = global write "DATA LOG.vi" "OP 40 reset"(w115) -> ()
      n55 = global write "DATA LOG.vi" "OP 60 reset"(w115) -> ()
      n56 = global write "DATA LOG.vi" "op 60"(0 ("op 30")) -> ()
      n57 = global write "DATA LOG.vi" "op 30"(0 ("op 30")) -> ()
      n58 = global write "DATA LOG.vi" "op 40"(0 ("op 30")) -> ()
    }
  }
  n59 = while {
    tunnel: w70 -> [w154]
    tunnel: w22 -> [w150]
    tunnel: w24 -> [w149]
    tunnel: w16 -> [w148]
    tunnel: [w123] -> w68
    tunnel: [w147] -> w67
    tunnel: FALSE -> [w146]
    tunnel: "REPORT" -> [w145]
    shift-right: [w143] -> _
    shift-left: string[] [] -> [w144]
    shift-right: [w142] -> _
    shift-left: "" ("trimmed string") -> [w141]
    shift-right: [w130] -> _
    shift-left: w3 -> [w139]
    stop <- w151 stop-if-true
    n60 = Dequeue Element(queue=w154, timeout in ms (-1)=250, error in (no error)=w150) -> (queue out=w126:refnum<queue>, element=w152:cluster{"CASE 2":T12}, error out=w153:errorcluster)  [unwired: 1 out]
    n61 = case shown="No Error" w153 {
      tunnel: w152 -> [w170 _]
      tunnel: [w166 TRUE] -> w151
      tunnel: w149 -> [w167 w1383]
      tunnel: w148 -> [w168 w1382]
      tunnel: [w164 w1383] -> w124
      tunnel: [w165 w1382] -> w147
      tunnel: w146 -> [w163 _]
      tunnel: w145 -> [w162 _]
      tunnel: w144 -> [w161 w1381]
      tunnel: [w160 w1381] -> w143
      tunnel: [w159 w1380] -> w142
      tunnel: w141 -> [w158 w1380]
      tunnel: w139 -> [w157 w1379]
      tunnel: [w156 w1379] -> w130
      tunnel: w126 -> [w155 _]
      frame No Error {
        n62 = Unbundle By Name(w170) -> ("CASE 2"=w169:T12)
        n63 = case shown="\"SCAN11\"" w169 {
          tunnel: w168 -> [w237 w261 w327 w397 w448 w509 w561 w610 w657 w714 w761 w815 w862 w927 w974 w1021 w1068 w1115 w1162 w1211 w1249 w1308 w1366 w1374]
          tunnel: w167 -> [w234 w257 w304 w396 w435 w508 w547 w609 w643 w713 w748 w814 w848 w926 w960 w1020 w1054 w1114 w1148 w1210 w1248 w1290 w1365 w1376]
          tunnel: [FALSE FALSE FALSE FALSE FALSE FALSE FALSE FALSE FALSE FALSE FALSE FALSE FALSE FALSE FALSE FALSE FALSE FALSE FALSE FALSE FALSE FALSE FALSE TRUE] -> w166
          tunnel: [w237 w259 w324 w394 w445 w506 w558 w607 w654 w711 w758 w812 w859 w924 w971 w1018 w1065 w1112 w1159 w1208 w1246 w1305 w1366 w1373] -> w165
          tunnel: [w172 w239 w323 w391 w430 w503 w542 w604 w638 w708 w743 w809 w843 w921 w955 w1015 w1049 w1109 w1143 w1205 w1243 w1289 w1365 w1375] -> w164
          tunnel: w163 -> [_ w254 w326 w393 w447 w505 w560 w606 w656 w710 w760 w811 w861 w923 w973 w1017 w1067 w1111 w1161 w1207 w1245 w1307 _ _]
          tunnel: w162 -> [_ w260 w325 w395 w446 w507 w559 w608 w655 w712 w759 w813 w860 w925 w972 w1019 w1066 w1113 w1160 w1209 w1247 w1306 _ _]
          tunnel: w161 -> [w236 w258 w320 w388 w444 w501 w557 w602 w653 w706 w757 w807 w858 w919 w970 w1013 w1064 w1107 w1158 w1203 w1241 w1304 w1363 w1377]
          tunnel: [w236 w258 w320 w388 w444 w501 w557 w602 w653 w706 w757 w807 w858 w919 w970 w1013 w1064 w1107 w1158 w1203 w1241 w1304 w1363 w1377] -> w160
          tunnel: [w235 w253 w316 w389 w440 w500 w553 w601 w649 w705 w753 w806 w854 w918 w966 w1012 w1060 w1106 w1154 w1202 w1240 w1300 w1362 w1368] -> w159
          tunnel: w158 -> [w235 w253 w316 w389 w440 w500 w553 w601 w649 w705 w753 w806 w854 w918 w966 w1012 w1060 w1106 w1154 w1202 w1240 w1300 w1362 w1368]
          tunnel: w157 -> [w233 w247 w314 w387 w429 w499 w551 w600 w647 w704 w742 w805 w852 w917 w964 w1011 w1058 w1105 w1152 w1201 w1239 w1298 w1361 w1367]
          tunnel: [w174 w247 w314 w387 w429 w499 w551 w600 w647 w704 w742 w805 w852 w917 w964 w1011 w1058 w1105 w1152 w1201 w1239 w1298 w1361 w1367] -> w156
          tunnel: w155 -> [_ w241 _ _ _ _ _ _ _ _ _ _ _ _ _ _ _ _ _ _ _ _ _ _]
          frame "-1", Default {
            n64 = control-ref of="Final Result"() -> (w224:refnum<vi>)
            n65 = control-ref of="Top Result"() -> (w228:refnum<vi>)
            n66 = control-ref of="Bottom Result"() -> (w230:refnum<vi>)
            n67 = control-ref of="Camera Status"() -> (w229:refnum<vi>)
            n68 = control-ref of="Camera Status"() -> (w227:refnum<vi>)
            n69 = control-ref of="Final Result"() -> (w226:refnum<vi>)
            n70 = control-ref of="Final Result"() -> (w220:refnum<vi>)
            n71 = control-ref of="Shaft Status"() -> (w221:refnum<vi>)
            n72 = call "OP10 Indicators.vi"("error in (no error)"=w234, "OUTPUT INDICATOR in"=w233, "Boolean in"=w224) -> ("error out"=w223:errorcluster, "OUTPUT INDICATOR out"=w232:T11)  [unwired: 7 in]
            n73 = Build Array(w230, w229, w228, w227, w226) -> (w225:refnum<vi>[])
            n74 = Build Array(w221, w220) -> (w219:refnum<vi>[])
            n75 = control-ref of="RH Status"() -> (w216:refnum<vi>)
            n76 = control-ref of="LH Status"() -> (w215:refnum<vi>)
            n77 = control-ref of="Final Result"() -> (w214:refnum<vi>)
            n78 = call "OP20 Indicators.vi"("error in (no error)"=w223, "Array"=w225, "OUTPUT INDICATOR in"=w232) -> ("error out"=w222:errorcluster, "OUTPUT INDICATOR out"=w231:T11)  [unwired: 7 in]
            n79 = control-ref of="Nut Status"() -> (w210:refnum<vi>)
            n80 = control-ref of="RH Status"() -> (w209:refnum<vi>)
            n81 = control-ref of="LH Status"() -> (w208:refnum<vi>)
            n82 = control-ref of="Camera Status"() -> (w207:refnum<vi>)
            n83 = control-ref of="Final Result"() -> (w206:refnum<vi>)
            n84 = Build Array(w216, w215, w214) -> (w213:refnum<vi>[])
            n85 = call "OP30 Indicators.vi"("error in (no error)"=w222, "Array"=w219, "OUTPUT INDICATOR in"=w231) -> ("error out"=w217:errorcluster, "OUTPUT INDICATOR out"=w218:T11)  [unwired: 7 in]
            n86 = Build Array(w210, w209, w208, w207, w206) -> (w205:refnum<vi>[])
            n87 = call "OP40 Indicators.vi"("error in (no error)"=w217, "Array"=w213, "OUTPUT INDICATOR in"=w218) -> ("error out"=w212:errorcluster, "OUTPUT INDICATOR out"=w211:T11)  [unwired: 7 in]
            n88 = control-ref of="Screw 1 Status"() -> (w201:refnum<vi>)
            n89 = control-ref of="Screw 2 Status"() -> (w200:refnum<vi>)
            n90 = control-ref of="Screw 3 Status"() -> (w199:refnum<vi>)
            n91 = control-ref of="Screw 4 Status"() -> (w198:refnum<vi>)
            n92 = control-ref of="Screw 5 Status"() -> (w197:refnum<vi>)
            n93 = control-ref of="Screw 6 Status"() -> (w196:refnum<vi>)
            n94 = control-ref of="Final Result"() -> (w195:refnum<vi>)
            n95 = control-ref of="Final Result"() -> (w192:refnum<vi>)
            n96 = call "OP50 Indicators.vi"("error in (no error)"=w212, "Array"=w205, "OUTPUT INDICATOR in"=w211) -> ("error out"=w204:errorcluster, "OUTPUT INDICATOR out"=w203:T11)  [unwired: 7 in]
            n97 = Build Array(w201, w200, w199, w198, w197, w196, w195) -> (w202:refnum<vi>[])
            n98 = control-ref of="Loctite Status"() -> (w188:refnum<vi>)
            n99 = control-ref of="Final Result"() -> (w187:refnum<vi>)
            n100 = Build Array(w192) -> (w191:refnum<vi>[])
            n101 = call "OP60 Indicators.vi"("error in (no error)"=w204, "Array"=w202, "OUTPUT INDICATOR in"=w203) -> ("error out"=w194:errorcluster, "OUTPUT INDICATOR out"=w193:T11)  [unwired: 7 in]
            n102 = call "OP70 Indicators.vi"("error in (no error)"=w194, "Array"=w191, "OUTPUT INDICATOR in"=w193) -> ("error out"=w190:errorcluster, "OUTPUT INDICATOR out"=w189:T11)  [unwired: 7 in]
            n103 = control-ref of="Seat Status"() -> (w183:refnum<vi>)
            n104 = control-ref of="Final Result"() -> (w182:refnum<vi>)
            n105 = control-ref of="Final Result"() -> (w178:refnum<vi>)
            n106 = Build Array(w188, w187) -> (w186:refnum<vi>[])
            n107 = call "OP80 Indicators.vi"("error in (no error)"=w190, "Array"=w186, "OUTPUT INDICATOR in"=w189) -> ("error out"=w184:errorcluster, "OUTPUT INDICATOR out"=w185:T11)  [unwired: 7 in]
            n108 = Build Array(w183, w182) -> (w181:refnum<vi>[])
            n109 = Build Array(w178) -> (w177:refnum<vi>[])
            n110 = call "OP90 Indicators.vi"("error in (no error)"=w184, "Array"=w181, "OUTPUT INDICATOR in"=w185) -> ("error out"=w180:errorcluster, "OUTPUT INDICATOR out"=w179:T11)  [unwired: 7 in]
            n111 = call "OP100 Indicators.vi"("error in (no error)"=w180, "Array"=w177, "OUTPUT INDICATOR in"=w179) -> ("error out"=w172:errorcluster, "OUTPUT INDICATOR out"=w175:T11)  [unwired: 7 in]
            n112 = call "PADMINI_AUTO_BARCODE_STRING 100.vi"("Enum"=enum16{"Read", "Write"}."Read", "error in (no error)"=w172) -> ("Input 2"=w173:string[])  [unwired: 8 in, 1 out]
            n113 = Index Array(array=w173) -> (element=w171:string)  [unwired: 1 in]
            n114 = Bundle By Name(cluster=w175, "OP - 110.BARCODE"=w171) -> (w174:T11)
          }
          frame "SCAN1" {
            # "STATION OP 10"
            n115 = global read "Global 1.vi" "BARCODE RECIPE"() -> (w248:string)
            n116 = call "PADMINI_AUTO_BARCODE_STRING.vi"("Enum"=enum16{"Read", "Write"}."Read", "error in (no error)"=w257) -> ("error out"=w256:errorcluster, "Input 2"=w244:string[])  [unwired: 8 in]
            n117 = Index Array(array=w244) -> (element=w243:string)  [unwired: 1 in]
            n118 = call <vilib>:"Trim Whitespace.vi"("string"=w243) -> ("trimmed string"=w242:string)  [unwired: 1 in]
            n119 = Match Pattern(string=w242, regular expression=w248) -> (match substring=w251:string)  [unwired: 1 in, 3 out]
            n120 = String Length(string=w248) -> (length=w250:i32)
            n121 = String Length(string=w251) -> (length=w249:i32)
            n122 = Equal?(x=w250, y=w249) -> (x = y?=w255:bool)
            n123 = case shown="False" w254 {
              tunnel: w261 -> [w285 w303]
              tunnel: w256 -> [w284 w301]
              tunnel: w260 -> [w283 _]
              tunnel: [w282 w300] -> w246
              tunnel: [w281 w303] -> w259
              tunnel: w255 -> [_ _]
              tunnel: w242 -> [w280 _]
              tunnel: [w279 TRUE] -> w240
              frame False {
                n124 = Format Into String(format string="where BARCODE='%s'", w280) -> (resulting string=w276:string)  [unwired: 2 in, 1 out]
                n125 = call <vilib>:"DB Tools Select Data.vi"("condition"=w276, "error in (no error)"=w284, "columns"=string[] ["BARCODE", "OP10_FINAL_RST"], "table"=w283, "connection reference"=w285) -> ("error out"=w275:errorcluster, "data"=w274:variant[][], "connection reference out"=w281:T13)  [unwired: 1 in]
                n126 = call "PADMINI_varient_to_data.vi"("error in (no error)"=w275, "data"=w274) -> ("error out"=w272:errorcluster, "Array"=w271:string[][])  [unwired: 8 in]
                n127 = Index Array(array=w271, index (row)=0, index (col)=1 ("index (row)")) -> (element=w268:string)
                n128 = Empty Array?(array=w271) -> (empty?=w273:bool)
                n129 = case shown="False" w273 {
                  tunnel: w272 -> [w295 w297]
                  tunnel: [w294 w297] -> w282
                  tunnel: [FALSE TRUE] -> w279
                  tunnel: w268 -> [w288 _]
                  frame False {
                    w287 = "OK"  # y
                    w290 = i32[] [1, 0]  # I/P
                    w289 = i32[] [0, 1]  # I/P
                    # "OP10 CURRENT STATION OK-NG\nPART REPEAT"
                    n130 = Equal?(x=w288, y=w287) -> (x = y?=w286:bool)
                    n131 = Select(t=w290, s=w286, f=w289) -> (s? t:f=w291:i32[])
                    n132 = call "PADMINI_AUTO_BARCODE_STATUS.vi"("Enum"=enum16{"Read", "Write"}."Write", "error in (no error)"=w295, "I/P"=w291) -> ("error out"=w294:errorcluster)  [unwired: 7 in, 1 out]
                  }
                  frame True {
                    # "OP10 NEW part"
                  }
                }
              }
              frame True {
                w299 = i32[] [0, 1]  # I/P
                n133 = call "PADMINI_AUTO_BARCODE_STATUS.vi"("Enum"=enum16{"Read", "Write"}."Write", "error in (no error)"=w301, "I/P"=w299) -> ("error out"=w300:errorcluster)  [unwired: 7 in, 1 out]
              }
            }
            n134 = flat-sequence {
              tunnel: [w267] -> w245
              tunnel: w246 -> [w267]
              frame #0 {
                # "UPDATE op 10 sCAN sTATUS"
                n135 = global write "DATA LOG.vi" "OP 10 Outputs"(TRUE) -> ()
              }
            }
            n136 = call <vilib>:"Clear Errors.vi"("error in (no error)"=w245) -> ("error out"=w239:errorcluster)  [unwired: 5 in, 1 out]
            n137 = case shown="True" w240 {
              tunnel: w241 -> [_ w265]
              tunnel: w239 -> [_ w263]
              frame False {
              }
              frame True {
                w264 = cluster{"CASE 2":T12} {"CASE 2"=enum."DATALOG1"}  # element
                n138 = Enqueue Element(queue=w265, element=w264, error in (no error)=w263) -> ()  [unwired: 1 in, 3 out]
              }
            }
          }
          frame "DATALOG1" {
            w318 = T14 2 items=["no dialog", "OK message", "continue or stop message", "OK message + warnings", "continue/stop + warnings"] ("type of dialog (OK msg:1)")
            # "cycle result status\nwhether it was ok or nok\nor abortted in between"
            # "Printed QR Code data string"
            # "datalog of OP 10"
            n139 = call "PADMINI_AUTO_BARCODE_STRING.vi"("Enum"=enum16{"Read", "Write"}."Read", "error in (no error)"=w304) -> ("Input 2"=w311:string[])  [unwired: 8 in, 1 out]
            n140 = call "PADMINI_AUTO_CYCLE VALUE 10.vi"("Enum"=enum16{"Read", "Write"}."Read", "error in (no error)"=w304) -> ("error out"=w307:errorcluster, "Input 2"=w306:sgl[])  [unwired: 8 in]
            n141 = Index Array(array=w306) -> (element=w305:sgl)  [unwired: 1 in]
            n142 = Index Array(array=w311) -> (element #1=w310:string, element #2=w309:string)  [unwired: 2 in]
            n143 = Number To Fractional String(number=w305, precision (6)=i16 2) -> (F-format string=w312:string)  [unwired: 2 in]
            n144 = call <vilib>:"Trim Whitespace.vi"("string"=w310) -> ("trimmed string"=w321:string)  [unwired: 1 in]
            n145 = case shown="False" w326 {
              tunnel: w327 -> [w351 w386]
              tunnel: w307 -> [w353 w385]
              tunnel: [w359 w384] -> w324
              tunnel: [w358 w383] -> w319
              tunnel: w325 -> [w348 _]
              tunnel: w321 -> [w345 _]
              tunnel: w309 -> [w355 w376]
              tunnel: w312 -> [w339 w375]
              frame False {
                w347 = string[] ["BARCODE", "SHIFT", "DATE", "OP10_LEAK_RATE", "OP10_FINAL_RST"]
                # "ST1 RESULT"
                # "DO TRACEBILITY"
                n146 = local read "SHIFT"() -> (w357:string)
                n147 = Format Into String(format string="Where BARCODE='%s' ", w345) -> (resulting string=w340:string)  [unwired: 2 in, 1 out]
                n148 = call <vilib>:"DB Tools Select Data.vi"("condition"=w340, "error in (no error)"=w353, "columns"=w347, "table"=w348, "connection reference"=w351) -> ("error out"=w349:errorcluster, "data"=w352:variant[][], "connection reference out"=w350:T13)  [unwired: 1 in]
                n149 = call "PADMINI_SHIFT_DATE.vi"("SHIFT"=w357) -> ("date/time string"=w356:string)  [unwired: 10 in]
                n150 = Variant To Data(error in=w349, type=string[][] [], Variant=w352) -> (data=w343:string[][], error out=w341:errorcluster)
                n151 = Bundle("trimmed string"=w345, "SHIFT"=w357, "date/time string"=w356, w339, "Input 2"=w355) -> (w354:T15)  [unwired: 1 in]
                n152 = Empty Array?(array=w343) -> (empty?=w342:bool)
                n153 = case shown="False" w342 {
                  tunnel: w350 -> [w364 w374]
                  tunnel: w341 -> [w363 w373]
                  tunnel: [w367 w372] -> w359
                  tunnel: [w366 w371] -> w358
                  tunnel: w347 -> [w361 w370]
                  tunnel: w348 -> [w362 w369]
                  tunnel: w354 -> [w365 w368]
                  tunnel: w340 -> [w360 _]
                  frame False {
                    n154 = call <vilib>:"DB Tools Update Data.vi"("condition"=w360, "data"=w365, "error in (no error)"=w363, "columns"=w361, "table"=w362, "connection reference"=w364) -> ("error out"=w366:errorcluster, "connection reference out"=w367:T13)  [unwired: 4 in]
                  }
                  frame True {
                    n155 = call <vilib>:"DB Tools Insert Data.vi"("data"=w368, "error in (no error)"=w373, "columns"=w370, "table"=w369, "connection reference"=w374) -> ("error out"=w371:errorcluster, "connection reference out"=w372:T13)  [unwired: 5 in]
                  }
                }
              }
              frame True {
                # "Trac BYPASS"
                n156 = local read "SHIFT"() -> (w381:string)
                n157 = call "PADMINI_SHIFT_DATE.vi"("SHIFT"=w381) -> ("date/time string"=w380:string)  [unwired: 10 in]
                n158 = Bundle("SHIFT"=w381, "date/time string"=w380, "Input 2"=w376, w375) -> (w379:T16)  [unwired: 1 in]
                n159 = To Variant(anything=w379) -> (Variant=w378:variant)
                n160 = call <vilib>:"DB Tools Insert Data.vi"("data"=w378, "error in (no error)"=w385, "columns"=string[] ["DATE", "SHIFT", "OP10_LEAK_RAT", "OP10_FINAL_RST"], "table"="ST1_REPORT", "connection reference"=w386) -> ("error out"=w383:errorcluster, "connection reference out"=w384:T13)  [unwired: 5 in]
              }
            }
            n161 = call <vilib>:"Simple Error Handler.vi"("type of dialog (OK msg:1)"=w318, "error in (no error)"=w319) -> ("error out"=w317:errorcluster)  [unwired: 3 in, 4 out]
            n162 = call <vilib>:"Clear Errors.vi"("error in (no error)"=w317) -> ("error out"=w315:errorcluster)  [unwired: 5 in, 1 out]
            n163 = disable-structure shown="Enabled" {
              disable-tunnel: [w337 w338] -> w323
              disable-tunnel: w315 -> [w336 w338]
              frame Disabled {
                w331 = refnum<vi> refnum  # Boolean
                n164 = property on="OP - 10" class="Clust"(error in=w336) -> (error out=w330:errorcluster, "Controls[]"=w334:refnum<vi>[])  [unwired: 1 in, 1 out]
                n165 = Index Array(array=w334, index=2) -> (element=w332:refnum<vi>)
                n166 = To More Specific Class(target class=w331, reference=w332, error in=w330) -> (specific class reference=w335:refnum<vi>, error out=w329:errorcluster)
                n167 = call "PADMINI_BOOL_COLOR_CHANGE.vi"("error in (no error)"=w329, "Boolean in"=w335) -> ("error out"=w337:errorcluster)  [unwired: 9 in]
              }
              frame Enabled {
              }
            }
          }
          frame "SCAN2" {
            # "Barcode Status\n0-Ideal, 1-Ok, 2-Nok, 3-Prev Station Not Done,\n4-Prev Station Nok,\n5- Already Done"
            # "STATION OP 20"
            n168 = case shown="False" w393 {
              tunnel: w397 -> [w420 w426]
              tunnel: w396 -> [w413 w424]
              tunnel: w395 -> [w401 _]
              tunnel: [w415 w423] -> w392
              tunnel: [w414 w426] -> w394
              tunnel: [w402 "" ("trimmed string")] -> _
              frame False {
                # "ST2 RESULT"
                # "ST1 RESULT"
                # "2 FOR EMPTY BARCODE READ OR MISMATCH"
                n169 = call "PADMINI_AUTO_BARCODE_STRING2.vi"("Enum"=enum16{"Read", "Write"}."Read", "error in (no error)"=w413) -> ("error out"=w412:errorcluster, "Input 2"=w404:string[])  [unwired: 8 in]
                n170 = global read "Global 1.vi" "BARCODE RECIPE"() -> (w405:string)
                n171 = Index Array(array=w404) -> (element=w403:string)  [unwired: 1 in]
                n172 = call <vilib>:"Trim Whitespace.vi"("string"=w403) -> ("trimmed string"=w402:string)  [unwired: 1 in]
                n173 = Match Pattern(string=w402, regular expression=w405) -> (match substring=w406:string)  [unwired: 1 in, 3 out]
                n174 = String Length(string=w405) -> (length=w408:i32)
                n175 = String Length(string=w406) -> (length=w407:i32)
                n176 = Format Into String(format string="WHERE BARCODE  ='%s'", w402) -> (resulting string=w409:string)  [unwired: 2 in, 1 out]
                n177 = Equal?(x=w408, y=w407) -> ()  [unwired: 1 out]
                n178 = call <vilib>:"DB Tools Select Data.vi"("condition"=w409, "error in (no error)"=w412, "columns"=string[] ["BARCODE", "OP10_FINAL_RST", "OP20_FINAL_RST"], "table"=w401, "connection reference"=w420) -> ("error out"=w418:errorcluster, "data"=w417:variant[][], "connection reference out"=w414:T13)  [unwired: 1 in]
                n179 = call "PADMINI_varient_to_data.vi"("error in (no error)"=w418, "data"=w417) -> ("error out"=w416:errorcluster, "Array"=w400:string[][])  [unwired: 8 in]
                n180 = call "RESPONSE_LOGIC.vi"("Array"=w400) -> ("Not Found"=w398:i32[])  [unwired: 10 in]
                n181 = call "PADMINI_AUTO_BARCODE_STATUS 20.vi"("Enum"=enum16{"Read", "Write"}."Write", "error in (no error)"=w416, "I/P"=w398) -> ("error out"=w415:errorcluster)  [unwired: 7 in, 1 out]
              }
              frame True {
                w421 = i32[] [0, 0, 0, 0, 0]  # I/P
                n182 = call "PADMINI_AUTO_BARCODE_STATUS 20.vi"("Enum"=enum16{"Read", "Write"}."Write", "error in (no error)"=w424, "I/P"=w421) -> ("error out"=w423:errorcluster)  [unwired: 7 in, 1 out]
              }
            }
            n183 = flat-sequence {
              tunnel: [w428] -> w391
              tunnel: w392 -> [w428]
              frame #0 {
                # "UPDATE op 20 SCAN sTATUS"
                n184 = global write "DATA LOG.vi" "OP 20 Outputs"(TRUE) -> ()
              }
            }
          }
          frame "DATALOG2" {
            w442 = T14 2 items=["no dialog", "OK message", "continue or stop message", "OK message + warnings", "continue/stop + warnings"] ("type of dialog (OK msg:1)")
            # "Printed QR Code data string"
            # "datalog of OP 20"
            n185 = call "PADMINI_AUTO_BARCODE_STRING2.vi"("Enum"=enum16{"Read", "Write"}."Read", "error in (no error)"=w435) -> ("error out"=w437:errorcluster, "Input 2"=w431:string[])  [unwired: 8 in]
            n186 = call "PADMINI_AUTO_CYCLE VALUE 20.vi"("Enum"=enum16{"Read", "Write"}."Read", "error in (no error)"=w435) -> ("Input 2"=w433:sgl[])  [unwired: 8 in, 1 out]
            n187 = Number To Fractional String(number=w433, precision (6)=i16 2) -> (F-format string=w432:string[])  [unwired: 2 in]
            n188 = case shown="False" w447 {
              tunnel: w448 -> [w472 w498]
              tunnel: w437 -> [w473 w497]
              tunnel: [w476 w496] -> w445
              tunnel: [w475 w495] -> w443
              tunnel: w446 -> [w471 _]
              tunnel: w432 -> [w467 w480]
              tunnel: w431 -> [w459 w481]
              frame False {
                # "ST2 RESULT"
                # "DO TRACEBILITY"
                n189 = Index Array(array=w459) -> (element #1=w460:string, element #2=w458:string, element #3=w457:string, element #4=w456:string, element #5=w455:string, element #6=w454:string, element #7=w453:string)  [unwired: 7 in]
                n190 = local read "SHIFT"() -> (w474:string)
                n191 = Index Array(array=w467) -> (element #1=w466:string, element #2=w465:string, element #3=w464:string, element #4=w463:string)  [unwired: 4 in]
                n192 = call <vilib>:"Trim Whitespace.vi"("string"=w460) -> ("trimmed string"=w461:string)  [unwired: 1 in]
                n193 = call "PADMINI_SHIFT_DATE.vi"("SHIFT"=w474) -> ("date/time string"=w452:string)  [unwired: 10 in]
                n194 = Format Into String(format string="Where BARCODE='%s' ", w461) -> (resulting string=w469:string)  [unwired: 2 in, 1 out]
                n195 = Bundle("date/time string"=w452, "Input 2"=w466, "Input 2"=w465, "Input 2"=w458, "Input 2"=w457, "Input 2"=w464, "Input 2"=w463, "Input 2"=w456, "Input 2"=w455, "Input 2"=w454, "Input 2"=w453) -> (w462:T17)  [unwired: 1 in]
                n196 = call <vilib>:"DB Tools Update Data.vi"("condition"=w469, "data"=w462, "error in (no error)"=w473, "columns"=string[] ["DATEST2", "OP20_LOWER_BEARING_DIS", "OP20_LOWER_BEARING_LOAD", "OP20_BOTTOM_CAMERA_STATUS", "OP20_LOWER_BEARING_RST", "OP20_UPPER_BEARING_DIS", "OP20_UPPER_BEARING_LOAD", "OP20_UPPER_SIM_STATUS", "OP20_UPPER_CAMERA_STATUS", "OP20_UPPER_BERAING_RST", "OP20_FINAL_RST"], "table"=w471, "connection reference"=w472) -> ("error out"=w475:errorcluster, "connection reference out"=w476:T13)  [unwired: 4 in]
              }
              frame True {
                n197 = local read "SHIFT"() -> (w478:string)
                n198 = Index Array(array=w481) -> (element #2=w487:string, element #3=w486:string, element #4=w485:string, element #5=w484:string, element #6=w483:string, element #7=w477:string)  [unwired: 7 in, 1 out]
                n199 = call "PADMINI_SHIFT_DATE.vi"("SHIFT"=w478) -> ("date/time string"=w479:string)  [unwired: 10 in]
                n200 = Index Array(array=w480) -> (element #1=w491:string, element #2=w490:string, element #3=w489:string, element #4=w488:string)  [unwired: 4 in]
                n201 = Bundle("date/time string"=w479, "SHIFT"=w478, "Input 2"=w491, "Input 2"=w490, "Input 2"=w487, "Input 2"=w486, "Input 2"=w489, "Input 2"=w488, "Input 2"=w485, "Input 2"=w484, "Input 2"=w483, "Input 2"=w477) -> (w482:T18)  [unwired: 1 in]
                n202 = To Variant(anything=w482) -> (Variant=w493:variant)
                n203 = call <vilib>:"DB Tools Insert Data.vi"("data"=w493, "error in (no error)"=w497, "columns"=string[] ["DATE", "SHIFT", "ST2_LOWER_BEARING_DIS", "ST2_LOWER_BEARING_LOAD", "ST2_BOTTOM_CAMERA_STATUS", "ST2_LOWER_BEARING_RST", "ST2_UPPER_BEARING_DIS", "ST2_UPPER_BEARING_LOAD", "ST2_UPPER_SIM_STATUS", "ST2_UPPER_CAMERA_STATUS", "ST2_UPPER_BERAING_RST", "ST2_FINAL_RST"], "table"="ST2_REPORT", "connection reference"=w498) -> ("error out"=w495:errorcluster, "connection reference out"=w496:T13)  [unwired: 5 in]
              }
            }
            n204 = call <vilib>:"Simple Error Handler.vi"("type of dialog (OK msg:1)"=w442, "error in (no error)"=w443) -> ("error out"=w441:errorcluster)  [unwired: 3 in, 4 out]
            n205 = call <vilib>:"Clear Errors.vi"("error in (no error)"=w441) -> ("error out"=w439:errorcluster)  [unwired: 5 in, 1 out]
            n206 = flat-sequence {
              tunnel: [w451] -> w430
              tunnel: w439 -> [w451]
              frame #0 {
                # "UPDATE op 20 save"
                n207 = global write "DATA LOG.vi" "OP 20 reset"(TRUE) -> ()
              }
            }
          }
          frame "SCAN3" {
            # "STATION OP 30"
            n208 = case shown="False" w505 {
              tunnel: w509 -> [w533 w539]
              tunnel: w508 -> [w526 w537]
              tunnel: w507 -> [w513 _]
              tunnel: [w528 w536] -> w504
              tunnel: [w527 w539] -> w506
              tunnel: [w514 "" ("trimmed string")] -> _
              frame False {
                n209 = call "PADMINI_AUTO_BARCODE_STRING 30.vi"("Enum"=enum16{"Read", "Write"}."Read", "error in (no error)"=w526) -> ("error out"=w525:errorcluster, "Input 2"=w516:string[])  [unwired: 8 in]
                n210 = global read "Global 1.vi" "BARCODE RECIPE"() -> (w517:string)
                n211 = Index Array(array=w516) -> (element=w515:string)  [unwired: 1 in]
                n212 = call <vilib>:"Trim Whitespace.vi"("string"=w515) -> ("trimmed string"=w514:string)  [unwired: 1 in]
                n213 = Match Pattern(string=w514, regular expression=w517) -> (match substring=w518:string)  [unwired: 1 in, 3 out]
                n214 = String Length(string=w517) -> (length=w520:i32)
                n215 = String Length(string=w518) -> (length=w519:i32)
                n216 = Equal?(x=w514, y="") -> ()  [unwired: 1 out]
                n217 = Format Into String(format string="WHERE BARCODE  ='%s'", w514) -> (resulting string=w522:string)  [unwired: 2 in, 1 out]
                n218 = Equal?(x=w520, y=w519) -> ()  [unwired: 1 out]
                n219 = call <vilib>:"DB Tools Select Data.vi"("condition"=w522, "error in (no error)"=w525, "columns"=string[] ["BARCODE", "OP20_FINAL_RST", "OP30_FINAL_RST"], "table"=w513, "connection reference"=w533) -> ("error out"=w531:errorcluster, "data"=w530:variant[][], "connection reference out"=w527:T13)  [unwired: 1 in]
                n220 = call "PADMINI_varient_to_data.vi"("error in (no error)"=w531, "data"=w530) -> ("error out"=w529:errorcluster, "Array"=w512:string[][])  [unwired: 8 in]
                n221 = call "RESPONSE_LOGIC.vi"("Array"=w512) -> ("Not Found"=w510:i32[])  [unwired: 10 in]
                n222 = call "PADMINI_AUTO_BARCODE_STATUS 30.vi"("Enum"=enum16{"Read", "Write"}."Write", "error in (no error)"=w529, "I/P"=w510) -> ("error out"=w528:errorcluster)  [unwired: 7 in, 1 out]
              }
              frame True {
                w534 = i32[] [0, 0, 0, 0, 0]  # I/P
                n223 = call "PADMINI_AUTO_BARCODE_STATUS 30.vi"("Enum"=enum16{"Read", "Write"}."Write", "error in (no error)"=w537, "I/P"=w534) -> ("error out"=w536:errorcluster)  [unwired: 7 in, 1 out]
              }
            }
            n224 = flat-sequence {
              tunnel: [w541] -> w503
              tunnel: w504 -> [w541]
              frame #0 {
                # "UPDATE op 30 SCAN sTATUS"
                n225 = global write "DATA LOG.vi" "OP 30 Outputs"(TRUE) -> ()
              }
            }
          }
          frame "DATALOG3" {
            w555 = T14 2 items=["no dialog", "OK message", "continue or stop message", "OK message + warnings", "continue/stop + warnings"] ("type of dialog (OK msg:1)")
            # "Printed QR Code data string"
            # "datalog of OP 30"
            n226 = call "PADMINI_AUTO_BARCODE_STRING 30.vi"("Enum"=enum16{"Read", "Write"}."Read", "error in (no error)"=w547) -> ("error out"=w549:errorcluster, "Input 2"=w543:string[])  [unwired: 8 in]
            n227 = call "PADMINI_AUTO_CYCLE VALUE 30.vi"("Enum"=enum16{"Read", "Write"}."Read", "error in (no error)"=w547) -> ("Input 2"=w545:sgl[])  [unwired: 8 in, 1 out]
            n228 = Number To Fractional String(number=w545, precision (6)=i16 2) -> (F-format string=w544:string[])  [unwired: 2 in]
            n229 = case shown="False" w560 {
              tunnel: w561 -> [w579 w599]
              tunnel: w549 -> [w580 w598]
              tunnel: [w583 w597] -> w558
              tunnel: [w582 w596] -> w556
              tunnel: w559 -> [w578 _]
              tunnel: w544 -> [w574 w584]
              tunnel: w543 -> [w568 w585]
              frame False {
                # "DO TRACEBILITY"
                n230 = Index Array(array=w568) -> (element #1=w569:string, element #2=w567:string, element #3=w566:string)  [unwired: 3 in]
                n231 = local read "SHIFT"() -> (w581:string)
                n232 = Index Array(array=w574) -> (element #1=w573:string, element #2=w572:string)  [unwired: 2 in]
                n233 = call <vilib>:"Trim Whitespace.vi"("string"=w569) -> ("trimmed string"=w570:string)  [unwired: 1 in]
                n234 = call "PADMINI_SHIFT_DATE.vi"("SHIFT"=w581) -> ("date/time string"=w565:string)  [unwired: 10 in]
                n235 = Format Into String(format string="Where BARCODE='%s' ", w570) -> (resulting string=w576:string)  [unwired: 2 in, 1 out]
                n236 = Bundle("date/time string"=w565, "Input 2"=w573, "Input 2"=w572, "Input 2"=w567, "Input 2"=w566) -> (w571:T19)  [unwired: 1 in]
                n237 = call <vilib>:"DB Tools Update Data.vi"("condition"=w576, "data"=w571, "error in (no error)"=w580, "columns"=string[] ["DATEST3", "OP30_DISPLACEMENT", "OP30_SHAFT_PRESS_LOAD", "OP30_SHAFT_STATUS", "OP30_FINAL_RST"], "table"=w578, "connection reference"=w579) -> ("error out"=w582:errorcluster, "connection reference out"=w583:T13)  [unwired: 4 in]
              }
              frame True {
                # "TRAC BYPASS"
                n238 = local read "SHIFT"() -> (w586:string)
                n239 = call "PADMINI_SHIFT_DATE.vi"("SHIFT"=w586) -> ("date/time string"=w587:string)  [unwired: 10 in]
                n240 = Index Array(array=w585) -> (element #2=w591:string, element #3=w590:string)  [unwired: 3 in, 1 out]
                n241 = Index Array(array=w584) -> (element #1=w593:string, element #2=w592:string)  [unwired: 2 in]
                n242 = Bundle("date/time string"=w587, "SHIFT"=w586, "Input 2"=w593, "Input 2"=w592, "Input 2"=w591, "Input 2"=w590) -> (w588:T20)  [unwired: 1 in]
                n243 = To Variant(anything=w588) -> (Variant=w589:variant)
                n244 = call <vilib>:"DB Tools Insert Data.vi"("data"=w589, "error in (no error)"=w598, "columns"=string[] ["DATE", "SHIFT", "ST3_DISPLACEMENT", "ST3_LOAD", "ST3_MIDDLE_GEAR_SHAFT_STATUS", "ST3_FINAL_RST"], "table"="ST3_REPORT", "connection reference"=w599) -> ("error out"=w596:errorcluster, "connection reference out"=w597:T13)  [unwired: 5 in]
              }
            }
            n245 = call <vilib>:"Simple Error Handler.vi"("type of dialog (OK msg:1)"=w555, "error in (no error)"=w556) -> ("error out"=w554:errorcluster)  [unwired: 3 in, 4 out]
            n246 = call <vilib>:"Clear Errors.vi"("error in (no error)"=w554) -> ("error out"=w552:errorcluster)  [unwired: 5 in, 1 out]
            n247 = flat-sequence {
              tunnel: [w564] -> w542
              tunnel: w552 -> [w564]
              frame #0 {
                # "UPDATE op 20 save"
                n248 = global write "DATA LOG.vi" "OP 30 reset"(TRUE) -> ()
              }
            }
          }
          frame "SCAN4" {
            # "STATION OP 40"
            n249 = case shown="False" w606 {
              tunnel: w610 -> [w629 w635]
              tunnel: w609 -> [w622 w634]
              tunnel: w608 -> [w613 _]
              tunnel: [w624 w633] -> w605
              tunnel: [w623 w635] -> w607
              tunnel: [w615 "" ("trimmed string")] -> _
              frame False {
                n250 = call "PADMINI_AUTO_BARCODE_STRING 40.vi"("Enum"=enum16{"Read", "Write"}."Read", "error in (no error)"=w622) -> ("error out"=w621:errorcluster, "Input 2"=w617:string[])  [unwired: 8 in]
                n251 = Index Array(array=w617) -> (element=w616:string)  [unwired: 1 in]
                n252 = call <vilib>:"Trim Whitespace.vi"("string"=w616) -> ("trimmed string"=w615:string)  [unwired: 1 in]
                n253 = Format Into String(format string="WHERE BARCODE  ='%s'", w615) -> (resulting string=w618:string)  [unwired: 2 in, 1 out]
                n254 = call <vilib>:"DB Tools Select Data.vi"("condition"=w618, "error in (no error)"=w621, "columns"=string[] ["BARCODE", "OP30_FINAL_RST", "OP40_FINAL_RST"], "table"=w613, "connection reference"=w629) -> ("error out"=w627:errorcluster, "data"=w626:variant[][], "connection reference out"=w623:T13)  [unwired: 1 in]
                n255 = call "PADMINI_varient_to_data.vi"("error in (no error)"=w627, "data"=w626) -> ("error out"=w625:errorcluster, "Array"=w614:string[][])  [unwired: 8 in]
                n256 = call "RESPONSE_LOGIC.vi"("Array"=w614) -> ("Not Found"=w611:i32[])  [unwired: 10 in]
                n257 = call "PADMINI_AUTO_BARCODE_STATUS 40.vi"("Enum"=enum16{"Read", "Write"}."Write", "error in (no error)"=w625, "I/P"=w611) -> ("error out"=w624:errorcluster)  [unwired: 7 in, 1 out]
              }
              frame True {
                w630 = i32[] [0, 0, 0, 0, 0]  # I/P
                n258 = call "PADMINI_AUTO_BARCODE_STATUS 40.vi"("Enum"=enum16{"Read", "Write"}."Write", "error in (no error)"=w634, "I/P"=w630) -> ("error out"=w633:errorcluster)  [unwired: 7 in, 1 out]
              }
            }
            n259 = flat-sequence {
              tunnel: [w637] -> w604
              tunnel: w605 -> [w637]
              frame #0 {
                # "UPDATE op 40 SCAN sTATUS"
                n260 = global write "DATA LOG.vi" "OP 40 Outputs"(TRUE) -> ()
              }
            }
          }
          frame "DATALOG4" {
            w651 = T14 2 items=["no dialog", "OK message", "continue or stop message", "OK message + warnings", "continue/stop + warnings"] ("type of dialog (OK msg:1)")
            # "datalog of OP 40"
            n261 = call "PADMINI_AUTO_BARCODE_STRING 40.vi"("Enum"=enum16{"Read", "Write"}."Read", "error in (no error)"=w643) -> ("error out"=w645:errorcluster, "Input 2"=w639:string[])  [unwired: 8 in]
            n262 = call "PADMINI_AUTO_CYCLE VALUE 40.vi"("Enum"=enum16{"Read", "Write"}."Read", "error in (no error)"=w643) -> ("Input 2"=w641:sgl[])  [unwired: 8 in, 1 out]
            n263 = Number To Fractional String(number=w641, precision (6)=i16 2) -> (F-format string=w640:string[])  [unwired: 2 in]
            n264 = case shown="False" w656 {
              tunnel: w657 -> [w679 w703]
              tunnel: w645 -> [w680 w702]
              tunnel: [w683 w701] -> w654
              tunnel: [w682 w700] -> w652
              tunnel: w655 -> [w678 _]
              tunnel: w640 -> [w674 w685]
              tunnel: w639 -> [w669 w684]
              frame False {
                # "DO TRACEBILITY"
                n265 = Index Array(array=w669) -> (element #1=w670:string, element #2=w665:string, element #3=w664:string, element #4=w663:string, element #5=w662:string)  [unwired: 5 in]
                n266 = local read "SHIFT"() -> (w681:string)
                n267 = Index Array(array=w674) -> (element #1=w673:string, element #2=w668:string, element #3=w667:string, element #4=w666:string)  [unwired: 4 in]
                n268 = call <vilib>:"Trim Whitespace.vi"("string"=w670) -> ("trimmed string"=w671:string)  [unwired: 1 in]
                n269 = call "PADMINI_SHIFT_DATE.vi"("SHIFT"=w681) -> ("date/time string"=w661:string)  [unwired: 10 in]
                n270 = Format Into String(format string="Where BARCODE='%s' ", w671) -> (resulting string=w676:string)  [unwired: 2 in, 1 out]
                n271 = Bundle("date/time string"=w661, "Input 2"=w673, "Input 2"=w665, "Input 2"=w668, "Input 2"=w664, "Input 2"=w667, "Input 2"=w666, "Input 2"=w662, "Input 2"=w663) -> (w672:T21)  [unwired: 1 in]
                n272 = call <vilib>:"DB Tools Update Data.vi"("condition"=w676, "data"=w672, "error in (no error)"=w680, "columns"=string[] ["DATEST4", "OP40_RH_SCREW", "OP40_RH_STATUS", "OP40_LH_SCREW", "OP40_LH_STATUS", "OP40_DISPLACEMENT", "OP40_STACK_LOAD", "OP40_TOP_BEARING_CAMERA_STAUS", "OP40_FINAL_RST"], "table"=w678, "connection reference"=w679) -> ("error out"=w682:errorcluster, "connection reference out"=w683:T13)  [unwired: 4 in]
              }
              frame True {
                # "TRAC BYPASS"
                n273 = local read "SHIFT"() -> (w686:string)
                n274 = Index Array(array=w684) -> (element #2=w694:string, element #3=w693:string, element #4=w692:string, element #5=w691:string)  [unwired: 5 in, 1 out]
                n275 = call "PADMINI_SHIFT_DATE.vi"("SHIFT"=w686) -> ("date/time string"=w687:string)  [unwired: 10 in]
                n276 = Index Array(array=w685) -> (element #1=w688:string, element #2=w697:string, element #3=w696:string, element #4=w695:string)  [unwired: 4 in]
                n277 = Bundle("date/time string"=w687, "SHIFT"=w686, "Input 2"=w688, "Input 2"=w694, "Input 2"=w697, "Input 2"=w693, "Input 2"=w696, "Input 2"=w695, "Input 2"=w691, "Input 2"=w692) -> (w690:T22)  [unwired: 1 in]
                n278 = To Variant(anything=w690) -> (Variant=w689:variant)
                n279 = call <vilib>:"DB Tools Insert Data.vi"("data"=w689, "error in (no error)"=w702, "columns"=string[] ["DATE", "SHIFT", "ST4_SCREW1_DATA", "ST4_SCREW1_STATUS", "ST4_SCREW2_DATA", "ST4_SCREW2_STATUS", "ST4_DISPLACEMENT", "ST4_LOAD", "ST4_TOP_BEARING_CAMERA_STAUS", "ST4_FINAL_RST"], "table"="ST4_REPORT", "connection reference"=w703) -> ("error out"=w700:errorcluster, "connection reference out"=w701:T13)  [unwired: 5 in]
              }
            }
            n280 = call <vilib>:"Simple Error Handler.vi"("type of dialog (OK msg:1)"=w651, "error in (no error)"=w652) -> ("error out"=w650:errorcluster)  [unwired: 3 in, 4 out]
            n281 = call <vilib>:"Clear Errors.vi"("error in (no error)"=w650) -> ("error out"=w648:errorcluster)  [unwired: 5 in, 1 out]
            n282 = flat-sequence {
              tunnel: [w660] -> w638
              tunnel: w648 -> [w660]
              frame #0 {
                # "UPDATE op 20 save"
                n283 = global write "DATA LOG.vi" "OP 40 reset"(TRUE) -> ()
              }
            }
          }
          frame "SCAN5" {
            # "STATION OP 50"
            n284 = case shown="False" w710 {
              tunnel: w714 -> [w733 w739]
              tunnel: w713 -> [w726 w738]
              tunnel: w712 -> [w717 _]
              tunnel: [w728 w737] -> w709
              tunnel: [w727 w739] -> w711
              tunnel: [w719 "" ("trimmed string")] -> _
              frame False {
                n285 = call "PADMINI_AUTO_BARCODE_STRING 50.vi"("Enum"=enum16{"Read", "Write"}."Read", "error in (no error)"=w726) -> ("error out"=w725:errorcluster, "Input 2"=w721:string[])  [unwired: 8 in]
                n286 = Index Array(array=w721) -> (element=w720:string)  [unwired: 1 in]
                n287 = call <vilib>:"Trim Whitespace.vi"("string"=w720) -> ("trimmed string"=w719:string)  [unwired: 1 in]
                n288 = Format Into String(format string="WHERE BARCODE  ='%s'", w719) -> (resulting string=w722:string)  [unwired: 2 in, 1 out]
                n289 = call <vilib>:"DB Tools Select Data.vi"("condition"=w722, "error in (no error)"=w725, "columns"=string[] ["BARCODE", "OP40_FINAL_RST", "OP50_FINAL_RST"], "table"=w717, "connection reference"=w733) -> ("error out"=w731:errorcluster, "data"=w730:variant[][], "connection reference out"=w727:T13)  [unwired: 1 in]
                n290 = call "PADMINI_varient_to_data.vi"("error in (no error)"=w731, "data"=w730) -> ("error out"=w729:errorcluster, "Array"=w718:string[][])  [unwired: 8 in]
                n291 = call "RESPONSE_LOGIC.vi"("Array"=w718) -> ("Not Found"=w715:i32[])  [unwired: 10 in]
                n292 = call "PADMINI_AUTO_BARCODE_STATUS 50.vi"("Enum"=enum16{"Read", "Write"}."Write", "error in (no error)"=w729, "I/P"=w715) -> ("error out"=w728:errorcluster)  [unwired: 7 in, 1 out]
              }
              frame True {
                w734 = i32[] [0, 0, 0, 0, 0]  # I/P
                n293 = call "PADMINI_AUTO_BARCODE_STATUS 50.vi"("Enum"=enum16{"Read", "Write"}."Write", "error in (no error)"=w738, "I/P"=w734) -> ("error out"=w737:errorcluster)  [unwired: 7 in, 1 out]
              }
            }
            n294 = flat-sequence {
              tunnel: [w741] -> w708
              tunnel: w709 -> [w741]
              frame #0 {
                # "UPDATE op 50 SCAN sTATUS"
                n295 = global write "DATA LOG.vi" "OP 50 Outputs"(TRUE) -> ()
              }
            }
          }
          frame "DATALOG5" {
            w755 = T14 2 items=["no dialog", "OK message", "continue or stop message", "OK message + warnings", "continue/stop + warnings"] ("type of dialog (OK msg:1)")
            # "datalog of OP 50"
            n296 = call "PADMINI_AUTO_BARCODE_STRING 50.vi"("Enum"=enum16{"Read", "Write"}."Read", "error in (no error)"=w748) -> ("error out"=w750:errorcluster, "Input 2"=w744:string[])  [unwired: 8 in]
            n297 = call "PADMINI_AUTO_CYCLE VALUE 50.vi"("Enum"=enum16{"Read", "Write"}."Read", "error in (no error)"=w748) -> ("Input 2"=w746:sgl[])  [unwired: 8 in, 1 out]
            n298 = Number To Fractional String(number=w746, precision (6)=i16 2) -> (F-format string=w745:string[])  [unwired: 2 in]
            n299 = case shown="False" w760 {
              tunnel: w761 -> [w782 w804]
              tunnel: w750 -> [w783 w803]
              tunnel: [w786 w802] -> w758
              tunnel: [w785 w801] -> w756
              tunnel: w759 -> [w781 _]
              tunnel: w745 -> [w777 w788]
              tunnel: w744 -> [w772 w787]
              frame False {
                # "DO TRACEBILITY"
                n300 = Index Array(array=w772) -> (element #1=w773:string, element #2=w769:string, element #3=w768:string, element #4=w767:string, element #5=w765:string)  [unwired: 5 in]
                n301 = local read "SHIFT"() -> (w784:string)
                n302 = Index Array(array=w777) -> (element #1=w776:string, element #2=w771:string, element #3=w770:string)  [unwired: 3 in]
                n303 = call <vilib>:"Trim Whitespace.vi"("string"=w773) -> ("trimmed string"=w774:string)  [unwired: 1 in]
                n304 = call "PADMINI_SHIFT_DATE.vi"("SHIFT"=w784) -> ("date/time string"=w766:string)  [unwired: 10 in]
                n305 = Format Into String(format string="Where BARCODE='%s' ", w774) -> (resulting string=w779:string)  [unwired: 2 in, 1 out]
                n306 = Bundle("date/time string"=w766, "Input 2"=w776, "Input 2"=w769, "Input 2"=w771, "Input 2"=w768, "Input 2"=w770, "Input 2"=w767, "Input 2"=w765) -> (w775:T23)  [unwired: 1 in]
                n307 = call <vilib>:"DB Tools Update Data.vi"("condition"=w779, "data"=w775, "error in (no error)"=w783, "columns"=string[] ["DATEST5", "OP50_NUT_TORQUE", "OP50_NUT_STATUS", "OP50_RH_STATUS", "OP50_RH_MOTOR_SCREW", "OP50_LH_STATUS", "OP50_LH_MOTOR_SCREW", "OP50_FINAL_RST"], "table"=w781, "connection reference"=w782) -> ("error out"=w785:errorcluster, "connection reference out"=w786:T13)  [unwired: 4 in]
              }
              frame True {
                # "TRAC BYPASS"
                n308 = local read "SHIFT"() -> (w789:string)
                n309 = Index Array(array=w787) -> (element #2=w793:string, element #3=w792:string, element #4=w797:string)  [unwired: 4 in, 1 out]
                n310 = Index Array(array=w788) -> (element #1=w796:string, element #2=w795:string, element #3=w794:string)  [unwired: 3 in]
                n311 = call "PADMINI_SHIFT_DATE.vi"("SHIFT"=w789) -> ("date/time string"=w790:string)  [unwired: 10 in]
                n312 = Bundle("date/time string"=w790, "SHIFT"=w789, "Input 2"=w796, "Input 2"=w793, "Input 2"=w795, "Input 2"=w792, "Input 2"=w794, "Input 2"=w797) -> (w791:T24)  [unwired: 1 in]
                n313 = To Variant(anything=w791) -> (Variant=w800:variant)
                n314 = call <vilib>:"DB Tools Insert Data.vi"("data"=w800, "error in (no error)"=w803, "columns"=string[] ["DATE", "SHIFT", "ST5_SCREW1_DATA", "ST5_SCREW1_STATUS", "ST5_SCREW2_DATA", "ST5_SCREW2_STATUS", "ST5_SCREW3_DATA", "ST5_FINAL_RST"], "table"="ST5_REPORT", "connection reference"=w804) -> ("error out"=w801:errorcluster, "connection reference out"=w802:T13)  [unwired: 5 in]
              }
            }
            n315 = call <vilib>:"Simple Error Handler.vi"("type of dialog (OK msg:1)"=w755, "error in (no error)"=w756) -> ("error out"=w754:errorcluster)  [unwired: 3 in, 4 out]
            n316 = call <vilib>:"Clear Errors.vi"("error in (no error)"=w754) -> ("error out"=w752:errorcluster)  [unwired: 5 in, 1 out]
            n317 = flat-sequence {
              tunnel: [w764] -> w743
              tunnel: w752 -> [w764]
              frame #0 {
                # "UPDATE op 20 save"
                n318 = global write "DATA LOG.vi" "OP 50 reset"(TRUE) -> ()
              }
            }
          }
          frame "SCAN6" {
            # "STATION OP 60"
            n319 = case shown="False" w811 {
              tunnel: w815 -> [w834 w840]
              tunnel: w814 -> [w827 w839]
              tunnel: w813 -> [_ _]
              tunnel: [w829 w838] -> w810
              tunnel: [w828 w840] -> w812
              tunnel: [w819 "" ("trimmed string")] -> _
              frame False {
                n320 = call "PADMINI_AUTO_BARCODE_STRING 60.vi"("Enum"=enum16{"Read", "Write"}."Read", "error in (no error)"=w827) -> ("error out"=w826:errorcluster, "Input 2"=w821:string[])  [unwired: 8 in]
                n321 = Index Array(array=w821) -> (element=w820:string)  [unwired: 1 in]
                n322 = call <vilib>:"Trim Whitespace.vi"("string"=w820) -> ("trimmed string"=w819:string)  [unwired: 1 in]
                n323 = Format Into String(format string="WHERE BARCODE  ='%s'", w819) -> (resulting string=w822:string)  [unwired: 2 in, 1 out]
                n324 = call <vilib>:"DB Tools Select Data.vi"("condition"=w822, "error in (no error)"=w826, "columns"=string[] ["BARCODE", "OP50_FINAL_RST", "OP60_FINAL_RST"], "table"="REPORT", "connection reference"=w834) -> ("error out"=w832:errorcluster, "data"=w831:variant[][], "connection reference out"=w828:T13)  [unwired: 1 in]
                n325 = call "PADMINI_varient_to_data.vi"("error in (no error)"=w832, "data"=w831) -> ("error out"=w830:errorcluster, "Array"=w818:string[][])  [unwired: 8 in]
                n326 = call "RESPONSE_LOGIC.vi"("Array"=w818) -> ("Not Found"=w816:i32[])  [unwired: 10 in]
                n327 = call "PADMINI_AUTO_BARCODE_STATUS 60.vi"("Enum"=enum16{"Read", "Write"}."Write", "error in (no error)"=w830, "I/P"=w816) -> ("error out"=w829:errorcluster)  [unwired: 7 in, 1 out]
              }
              frame True {
                w835 = i32[] [0, 0, 0, 0, 0]  # I/P
                n328 = call "PADMINI_AUTO_BARCODE_STATUS 60.vi"("Enum"=enum16{"Read", "Write"}."Write", "error in (no error)"=w839, "I/P"=w835) -> ("error out"=w838:errorcluster)  [unwired: 7 in, 1 out]
              }
            }
            n329 = flat-sequence {
              tunnel: [w842] -> w809
              tunnel: w810 -> [w842]
              frame #0 {
                # "UPDATE op 60 SCAN sTATUS"
                n330 = global write "DATA LOG.vi" "OP 60 Outputs"(TRUE) -> ()
              }
            }
          }
          frame "DATALOG6" {
            w856 = T14 2 items=["no dialog", "OK message", "continue or stop message", "OK message + warnings", "continue/stop + warnings"] ("type of dialog (OK msg:1)")
            # "datalog of OP 60"
            n331 = call "PADMINI_AUTO_BARCODE_STRING 60.vi"("Enum"=enum16{"Read", "Write"}."Read", "error in (no error)"=w848) -> ("error out"=w850:errorcluster, "Input 2"=w844:string[])  [unwired: 8 in]
            n332 = call "PADMINI_AUTO_CYCLE VALUE 60.vi"("Enum"=enum16{"Read", "Write"}."Read", "error in (no error)"=w848) -> ("Input 2"=w846:sgl[])  [unwired: 8 in, 1 out]
            n333 = Number To Fractional String(number=w846, precision (6)=i16 2) -> (F-format string=w845:string[])  [unwired: 2 in]
            n334 = case shown="False" w861 {
              tunnel: w862 -> [w888 w916]
              tunnel: w850 -> [w889 w915]
              tunnel: [w892 w914] -> w859
              tunnel: [w891 w913] -> w857
              tunnel: w860 -> [w887 _]
              tunnel: w845 -> [w883 w896]
              tunnel: w844 -> [w878 w895]
              frame False {
                # "DO TRACEBILITY"
                n335 = Index Array(array=w878) -> (element #1=w879:string, element #2=w875:string, element #3=w874:string, element #4=w873:string, element #5=w871:string, element #6=w868:string, element #7=w867:string)  [unwired: 7 in]
                n336 = local read "SHIFT"() -> (w890:string)
                n337 = Index Array(array=w883) -> (element #1=w882:string, element #2=w877:string, element #3=w876:string, element #4=w872:string, element #5=w870:string, element #6=w869:string)  [unwired: 6 in]
                n338 = call <vilib>:"Trim Whitespace.vi"("string"=w879) -> ("trimmed string"=w880:string)  [unwired: 1 in]
                n339 = call "PADMINI_SHIFT_DATE.vi"("SHIFT"=w890) -> ("date/time string"=w866:string)  [unwired: 10 in]
                n340 = Format Into String(format string="Where BARCODE='%s' ", w880) -> (resulting string=w885:string)  [unwired: 2 in, 1 out]
                n341 = Bundle("date/time string"=w866, "Input 2"=w882, "Input 2"=w875, "Input 2"=w877, "Input 2"=w874, "Input 2"=w876, "Input 2"=w873, "Input 2"=w872, "Input 2"=w871, "Input 2"=w870, "Input 2"=w869, "Input 2"=w868, "Input 2"=w867) -> (w881:T25)  [unwired: 1 in]
                n342 = call <vilib>:"DB Tools Update Data.vi"("condition"=w885, "data"=w881, "error in (no error)"=w889, "columns"=string[] ["DATEST6", "OP60_SCREW1_DATA", "OP60_SCREW1_STATUS", "OP60_SCREW2_DATA", "OP60_SCREW2_STATUS", "OP60_SCREW3_DATA", "OP60_SCREW3_STATUS", "OP60_SCREW4_DATA", "OP60_SCREW4_STATUS", "OP60_SCREW5_DATA", "OP60_SCREW5_STATUS", "OP60_SCREW6_DATA", "OP60_SCREW6_STATUS", "OP60_FINAL_RST"], "table"=w887, "connection reference"=w888) -> ("error out"=w891:errorcluster, "connection reference out"=w892:T13)  [unwired: 4 in]
              }
              frame True {
                # "TRAC BYPASS"
                n343 = local read "SHIFT"() -> (w893:string)
                n344 = call "PADMINI_SHIFT_DATE.vi"("SHIFT"=w893) -> ("date/time string"=w894:string)  [unwired: 10 in]
                n345 = Index Array(array=w895) -> (element #2=w904:string, element #3=w903:string, element #4=w902:string, element #5=w900:string, element #6=w908:string, element #7=w909:string)  [unwired: 7 in, 1 out]
                n346 = Index Array(array=w896) -> (element #1=w907:string, element #2=w906:string, element #3=w905:string, element #4=w901:string, element #5=w899:string, element #6=w898:string)  [unwired: 6 in]
                n347 = Bundle("date/time string"=w894, "SHIFT"=w893, "Input 2"=w907, "Input 2"=w904, "Input 2"=w906, "Input 2"=w903, "Input 2"=w905, "Input 2"=w902, "Input 2"=w901, "Input 2"=w900, "Input 2"=w899, "Input 2"=w898, "Input 2"=w908, "Input 2"=w909) -> (w897:T26)  [unwired: 1 in]
                n348 = To Variant(anything=w897) -> (Variant=w912:variant)
                n349 = call <vilib>:"DB Tools Insert Data.vi"("data"=w912, "error in (no error)"=w915, "columns"=string[] ["DATE", "SHIFT", "ST6_SCREW1_DATA", "ST6_SCREW1_STATUS", "ST6_SCREW2_DATA", "ST6_SCREW2_STATUS", "ST6_SCREW3_DATA", "ST6_SCREW3_STATUS", "ST6_SCREW4_DATA", "ST6_SCREW4_STATUS", "ST6_SCREW5_DATA", "ST6_SCREW5_STATUS", "ST6_SCREW6_DATA", "ST6_SCREW6_STATUS", "ST6_FINAL_RST"], "table"="ST6_REPORT", "connection reference"=w916) -> ("error out"=w913:errorcluster, "connection reference out"=w914:T13)  [unwired: 5 in]
              }
            }
            n350 = call <vilib>:"Simple Error Handler.vi"("type of dialog (OK msg:1)"=w856, "error in (no error)"=w857) -> ("error out"=w855:errorcluster)  [unwired: 3 in, 4 out]
            n351 = call <vilib>:"Clear Errors.vi"("error in (no error)"=w855) -> ("error out"=w853:errorcluster)  [unwired: 5 in, 1 out]
            n352 = flat-sequence {
              tunnel: [w865] -> w843
              tunnel: w853 -> [w865]
              frame #0 {
                # "UPDATE op 20 save"
                n353 = global write "DATA LOG.vi" "OP 60 reset"(TRUE) -> ()
              }
            }
          }
          frame "SCAN7" {
            # "STATION OP 70"
            n354 = case shown="False" w923 {
              tunnel: w927 -> [w946 w952]
              tunnel: w926 -> [w939 w951]
              tunnel: w925 -> [w931 _]
              tunnel: [w941 w950] -> w922
              tunnel: [w940 w952] -> w924
              tunnel: [w932 "" ("trimmed string")] -> _
              frame False {
                n355 = call "PADMINI_AUTO_BARCODE_STRING 70.vi"("Enum"=enum16{"Read", "Write"}."Read", "error in (no error)"=w939) -> ("error out"=w938:errorcluster, "Input 2"=w934:string[])  [unwired: 8 in]
                n356 = Index Array(array=w934) -> (element=w933:string)  [unwired: 1 in]
                n357 = call <vilib>:"Trim Whitespace.vi"("string"=w933) -> ("trimmed string"=w932:string)  [unwired: 1 in]
                n358 = Format Into String(format string="WHERE BARCODE  ='%s'", w932) -> (resulting string=w935:string)  [unwired: 2 in, 1 out]
                n359 = call <vilib>:"DB Tools Select Data.vi"("condition"=w935, "error in (no error)"=w938, "columns"=string[] ["BARCODE", "OP60_FINAL_RST", "OP70_FINAL_RST"], "table"=w931, "connection reference"=w946) -> ("error out"=w944:errorcluster, "data"=w943:variant[][], "connection reference out"=w940:T13)  [unwired: 1 in]
                n360 = call "PADMINI_varient_to_data.vi"("error in (no error)"=w944, "data"=w943) -> ("error out"=w942:errorcluster, "Array"=w930:string[][])  [unwired: 8 in]
                n361 = call "RESPONSE_LOGIC.vi"("Array"=w930) -> ("Not Found"=w928:i32[])  [unwired: 10 in]
                n362 = call "PADMINI_AUTO_BARCODE_STATUS 70.vi"("Enum"=enum16{"Read", "Write"}."Write", "error in (no error)"=w942, "I/P"=w928) -> ("error out"=w941:errorcluster)  [unwired: 7 in, 1 out]
              }
              frame True {
                w947 = i32[] [0, 0, 0, 0, 0]  # I/P
                n363 = call "PADMINI_AUTO_BARCODE_STATUS 70.vi"("Enum"=enum16{"Read", "Write"}."Write", "error in (no error)"=w951, "I/P"=w947) -> ("error out"=w950:errorcluster)  [unwired: 7 in, 1 out]
              }
            }
            n364 = flat-sequence {
              tunnel: [w954] -> w921
              tunnel: w922 -> [w954]
              frame #0 {
                # "UPDATE op 70 SCAN sTATUS"
                n365 = global write "DATA LOG.vi" "OP 70 Outputs"(TRUE) -> ()
              }
            }
          }
          frame "DATALOG7" {
            w968 = T14 2 items=["no dialog", "OK message", "continue or stop message", "OK message + warnings", "continue/stop + warnings"] ("type of dialog (OK msg:1)")
            # "datalog of OP 70"
            n366 = call "PADMINI_AUTO_BARCODE_STRING 70.vi"("Enum"=enum16{"Read", "Write"}."Read", "error in (no error)"=w960) -> ("error out"=w962:errorcluster, "Input 2"=w956:string[])  [unwired: 8 in]
            n367 = call "PADMINI_AUTO_CYCLE VALUE 70.vi"("Enum"=enum16{"Read", "Write"}."Read", "error in (no error)"=w960) -> ("Input 2"=w958:sgl[])  [unwired: 8 in, 1 out]
            n368 = Number To Fractional String(number=w958, precision (6)=i16 2) -> (F-format string=w957:string[])  [unwired: 2 in]
            n369 = case shown="False" w973 {
              tunnel: w974 -> [w992 w1010]
              tunnel: w962 -> [w993 w1009]
              tunnel: [w995 w1008] -> w971
              tunnel: [w994 w1007] -> w969
              tunnel: w972 -> [w991 _]
              tunnel: w957 -> [w987 w997]
              tunnel: w956 -> [w982 w996]
              frame False {
                # "DO TRACEBILITY"
                n370 = Index Array(array=w982) -> (element #1=w983:string, element #2=w981:string)  [unwired: 2 in]
                n371 = call <vilib>:"Trim Whitespace.vi"("string"=w983) -> ("trimmed string"=w984:string)  [unwired: 1 in]
                n372 = local read "SHIFT"() -> (w979:string)
                n373 = Index Array(array=w987) -> (element #1=w986:string, element #2=w980:string)  [unwired: 2 in]
                n374 = call "PADMINI_SHIFT_DATE.vi"("SHIFT"=w979) -> ("date/time string"=w978:string)  [unwired: 10 in]
                n375 = Bundle("date/time string"=w978, "Input 2"=w986, "Input 2"=w980, "Input 2"=w981) -> (w985:T27)  [unwired: 1 in]
                n376 = Format Into String(format string="Where BARCODE='%s' ", w984) -> (resulting string=w989:string)  [unwired: 2 in, 1 out]
                n377 = call <vilib>:"DB Tools Update Data.vi"("condition"=w989, "data"=w985, "error in (no error)"=w993, "columns"=string[] ["DATE_OP70", "OP70_FULL_OPEN", "OP70_FULL_CLOSE", "OP70_FINAL_RST"], "table"=w991, "connection reference"=w992) -> ("error out"=w994:errorcluster, "connection reference out"=w995:T13)  [unwired: 4 in]
              }
              frame True {
                # "TRAC BYPASS"
                n378 = local read "SHIFT"() -> (w998:string)
                n379 = call "PADMINI_SHIFT_DATE.vi"("SHIFT"=w998) -> ("date/time string"=w999:string)  [unwired: 10 in]
                n380 = Index Array(array=w996) -> (element #2=w1002:string)  [unwired: 2 in, 1 out]
                n381 = Index Array(array=w997) -> (element #1=w1003:string, element #2=w1001:string)  [unwired: 2 in]
                n382 = Bundle("date/time string"=w999, "SHIFT"=w998, "Input 2"=w1003, "Input 2"=w1001, "Input 2"=w1002) -> (w1000:T28)  [unwired: 1 in]
                n383 = To Variant(anything=w1000) -> (Variant=w1006:variant)
                n384 = call <vilib>:"DB Tools Insert Data.vi"("data"=w1006, "error in (no error)"=w1009, "columns"=string[] ["DATE_OP70", "SHIFT", "OP70_FULL_OPEN", "OP70_FULL_CLOSE", "OP70_FINAL_RST"], "table"="ST7_REPORT", "connection reference"=w1010) -> ("error out"=w1007:errorcluster, "connection reference out"=w1008:T13)  [unwired: 5 in]
              }
            }
            n385 = call <vilib>:"Simple Error Handler.vi"("type of dialog (OK msg:1)"=w968, "error in (no error)"=w969) -> ("error out"=w967:errorcluster)  [unwired: 3 in, 4 out]
            n386 = call <vilib>:"Clear Errors.vi"("error in (no error)"=w967) -> ("error out"=w965:errorcluster)  [unwired: 5 in, 1 out]
            n387 = flat-sequence {
              tunnel: [w977] -> w955
              tunnel: w965 -> [w977]
              frame #0 {
                # "UPDATE op 20 save"
                n388 = global write "DATA LOG.vi" "OP 70 reset"(TRUE) -> ()
              }
            }
          }
          frame "SCAN8" {
            # "STATION OP 80"
            n389 = case shown="False" w1017 {
              tunnel: w1021 -> [w1040 w1046]
              tunnel: w1020 -> [w1033 w1045]
              tunnel: w1019 -> [w1025 _]
              tunnel: [w1035 w1044] -> w1016
              tunnel: [w1034 w1046] -> w1018
              tunnel: [w1026 "" ("trimmed string")] -> _
              frame False {
                (unwired) "REPORT"
                n390 = call "PADMINI_AUTO_BARCODE_STRING 80.vi"("Enum"=enum16{"Read", "Write"}."Read", "error in (no error)"=w1033) -> ("error out"=w1032:errorcluster, "Input 2"=w1028:string[])  [unwired: 8 in]
                n391 = Index Array(array=w1028) -> (element=w1027:string)  [unwired: 1 in]
                n392 = call <vilib>:"Trim Whitespace.vi"("string"=w1027) -> ("trimmed string"=w1026:string)  [unwired: 1 in]
                n393 = Format Into String(format string="WHERE BARCODE  ='%s'", w1026) -> (resulting string=w1029:string)  [unwired: 2 in, 1 out]
                n394 = call <vilib>:"DB Tools Select Data.vi"("condition"=w1029, "error in (no error)"=w1032, "columns"=string[] ["BARCODE", "OP70_FINAL_RST", "OP80_FINAL_RST"], "table"=w1025, "connection reference"=w1040) -> ("error out"=w1038:errorcluster, "data"=w1037:variant[][], "connection reference out"=w1034:T13)  [unwired: 1 in]
                n395 = call "PADMINI_varient_to_data.vi"("error in (no error)"=w1038, "data"=w1037) -> ("error out"=w1036:errorcluster, "Array"=w1024:string[][])  [unwired: 8 in]
                n396 = call "RESPONSE_LOGIC.vi"("Array"=w1024) -> ("Not Found"=w1022:i32[])  [unwired: 10 in]
                n397 = call "PADMINI_AUTO_BARCODE_STATUS 80.vi"("Enum"=enum16{"Read", "Write"}."Write", "error in (no error)"=w1036, "I/P"=w1022) -> ("error out"=w1035:errorcluster)  [unwired: 7 in, 1 out]
              }
              frame True {
                w1041 = i32[] [0, 0, 0, 0, 0]  # I/P
                n398 = call "PADMINI_AUTO_BARCODE_STATUS 80.vi"("Enum"=enum16{"Read", "Write"}."Write", "error in (no error)"=w1045, "I/P"=w1041) -> ("error out"=w1044:errorcluster)  [unwired: 7 in, 1 out]
              }
            }
            n399 = flat-sequence {
              tunnel: [w1048] -> w1015
              tunnel: w1016 -> [w1048]
              frame #0 {
                # "UPDATE op 80 SCAN sTATUS"
                n400 = global write "DATA LOG.vi" "OP 80 Outputs"(TRUE) -> ()
              }
            }
          }
          frame "DATALOG8" {
            w1062 = T14 2 items=["no dialog", "OK message", "continue or stop message", "OK message + warnings", "continue/stop + warnings"] ("type of dialog (OK msg:1)")
            # "datalog of OP 80"
            n401 = call "PADMINI_AUTO_BARCODE_STRING 80.vi"("Enum"=enum16{"Read", "Write"}."Read", "error in (no error)"=w1054) -> ("error out"=w1056:errorcluster, "Input 2"=w1050:string[])  [unwired: 8 in]
            n402 = call "PADMINI_AUTO_CYCLE VALUE 80.vi"("Enum"=enum16{"Read", "Write"}."Read", "error in (no error)"=w1054) -> ("Input 2"=w1052:sgl[])  [unwired: 8 in, 1 out]
            n403 = Number To Fractional String(number=w1052, precision (6)=i16 2) -> (F-format string=w1051:string[])  [unwired: 2 in]
            n404 = case shown="False" w1067 {
              tunnel: w1068 -> [w1086 w1104]
              tunnel: w1056 -> [w1087 w1103]
              tunnel: [w1089 w1102] -> w1065
              tunnel: [w1088 w1101] -> w1063
              tunnel: w1066 -> [w1085 _]
              tunnel: w1051 -> [w1081 w1092]
              tunnel: w1050 -> [w1077 w1093]
              frame False {
                # "DO TRACEBILITY"
                n405 = Index Array(array=w1077) -> (element #1=w1078:string, element #2=w1076:string, element #3=w1075:string)  [unwired: 3 in]
                n406 = call <vilib>:"Trim Whitespace.vi"("string"=w1078) -> ("trimmed string"=w1079:string)  [unwired: 1 in]
                n407 = local read "SHIFT"() -> (w1073:string)
                n408 = Index Array(array=w1081) -> (element=w1074:string)  [unwired: 1 in]
                n409 = call "PADMINI_SHIFT_DATE.vi"("SHIFT"=w1073) -> ("date/time string"=w1072:string)  [unwired: 10 in]
                n410 = Bundle("date/time string"=w1072, "Input 2"=w1074, "Input 2"=w1076, "Input 2"=w1075) -> (w1080:T27)  [unwired: 1 in]
                n411 = Format Into String(format string="Where BARCODE='%s' ", w1079) -> (resulting string=w1083:string)  [unwired: 2 in, 1 out]
                n412 = call <vilib>:"DB Tools Update Data.vi"("condition"=w1083, "data"=w1080, "error in (no error)"=w1087, "columns"=string[] ["DATE_OP80", "OP80_LOCTITE_STATUS", "OP80_PLUG_PRESS_LOA", "OP80_FINAL_RST"], "table"=w1085, "connection reference"=w1086) -> ("error out"=w1088:errorcluster, "connection reference out"=w1089:T13)  [unwired: 4 in]
              }
              frame True {
                # "TRAC BYPASS"
                n413 = local read "SHIFT"() -> (w1090:string)
                n414 = call "PADMINI_SHIFT_DATE.vi"("SHIFT"=w1090) -> ("date/time string"=w1091:string)  [unwired: 10 in]
                n415 = Index Array(array=w1093) -> (element #2=w1097:string, element #3=w1096:string)  [unwired: 3 in, 1 out]
                n416 = Index Array(array=w1092) -> (element=w1095:string)  [unwired: 1 in]
                n417 = Bundle("date/time string"=w1091, "SHIFT"=w1090, "Input 2"=w1095, "Input 2"=w1097, "Input 2"=w1096) -> (w1094:T28)  [unwired: 1 in]
                n418 = To Variant(anything=w1094) -> (Variant=w1100:variant)
                n419 = call <vilib>:"DB Tools Insert Data.vi"("data"=w1100, "error in (no error)"=w1103, "columns"=string[] ["DATE", "SHIFT", "ST8_DISPENSING", "ST8_LOAD", "ST8_FINAL_RST"], "table"="ST8_REPORT", "connection reference"=w1104) -> ("error out"=w1101:errorcluster, "connection reference out"=w1102:T13)  [unwired: 5 in]
              }
            }
            n420 = call <vilib>:"Simple Error Handler.vi"("type of dialog (OK msg:1)"=w1062, "error in (no error)"=w1063) -> ("error out"=w1061:errorcluster)  [unwired: 3 in, 4 out]
            n421 = call <vilib>:"Clear Errors.vi"("error in (no error)"=w1061) -> ("error out"=w1059:errorcluster)  [unwired: 5 in, 1 out]
            n422 = flat-sequence {
              tunnel: [w1071] -> w1049
              tunnel: w1059 -> [w1071]
              frame #0 {
                # "UPDATE op 20 save"
                n423 = global write "DATA LOG.vi" "OP 80 reset"(TRUE) -> ()
              }
            }
          }
          frame "SCAN9" {
            # "STATION OP 90"
            n424 = case shown="False" w1111 {
              tunnel: w1115 -> [w1134 w1140]
              tunnel: w1114 -> [w1127 w1139]
              tunnel: w1113 -> [w1119 _]
              tunnel: [w1129 w1138] -> w1110
              tunnel: [w1128 w1140] -> w1112
              tunnel: [w1120 "" ("trimmed string")] -> _
              frame False {
                (unwired) "REPORT"
                n425 = call "PADMINI_AUTO_BARCODE_STRING 90.vi"("Enum"=enum16{"Read", "Write"}."Read", "error in (no error)"=w1127) -> ("error out"=w1126:errorcluster, "Input 2"=w1122:string[])  [unwired: 8 in]
                n426 = Index Array(array=w1122) -> (element=w1121:string)  [unwired: 1 in]
                n427 = call <vilib>:"Trim Whitespace.vi"("string"=w1121) -> ("trimmed string"=w1120:string)  [unwired: 1 in]
                n428 = Format Into String(format string="WHERE BARCODE  ='%s'", w1120) -> (resulting string=w1123:string)  [unwired: 2 in, 1 out]
                n429 = call <vilib>:"DB Tools Select Data.vi"("condition"=w1123, "error in (no error)"=w1126, "columns"=string[] ["BARCODE", "OP80_FINAL_RST", "OP90_FINAL_RST"], "table"=w1119, "connection reference"=w1134) -> ("error out"=w1132:errorcluster, "data"=w1131:variant[][], "connection reference out"=w1128:T13)  [unwired: 1 in]
                n430 = call "PADMINI_varient_to_data.vi"("error in (no error)"=w1132, "data"=w1131) -> ("error out"=w1130:errorcluster, "Array"=w1118:string[][])  [unwired: 8 in]
                n431 = call "RESPONSE_LOGIC.vi"("Array"=w1118) -> ("Not Found"=w1116:i32[])  [unwired: 10 in]
                n432 = call "PADMINI_AUTO_BARCODE_STATUS 90.vi"("Enum"=enum16{"Read", "Write"}."Write", "error in (no error)"=w1130, "I/P"=w1116) -> ("error out"=w1129:errorcluster)  [unwired: 7 in, 1 out]
              }
              frame True {
                w1135 = i32[] [0, 0, 0, 0, 0]  # I/P
                n433 = call "PADMINI_AUTO_BARCODE_STATUS 90.vi"("Enum"=enum16{"Read", "Write"}."Write", "error in (no error)"=w1139, "I/P"=w1135) -> ("error out"=w1138:errorcluster)  [unwired: 7 in, 1 out]
              }
            }
            n434 = flat-sequence {
              tunnel: [w1142] -> w1109
              tunnel: w1110 -> [w1142]
              frame #0 {
                # "UPDATE op 90 SCAN sTATUS"
                n435 = global write "DATA LOG.vi" "OP 90 Outputs"(TRUE) -> ()
              }
            }
          }
          frame "DATALOG9" {
            w1156 = T14 2 items=["no dialog", "OK message", "continue or stop message", "OK message + warnings", "continue/stop + warnings"] ("type of dialog (OK msg:1)")
            # "datalog of OP 90"
            n436 = call "PADMINI_AUTO_BARCODE_STRING 90.vi"("Enum"=enum16{"Read", "Write"}."Read", "error in (no error)"=w1148) -> ("error out"=w1150:errorcluster, "Input 2"=w1145:string[])  [unwired: 8 in]
            n437 = call "PADMINI_AUTO_CYCLE VALUE 90.vi"("Enum"=enum16{"Read", "Write"}."Read", "error in (no error)"=w1148) -> ("Input 2"=w1144:sgl[])  [unwired: 8 in, 1 out]
            n438 = Number To Fractional String(number=w1144, precision (6)=i16 2) -> (F-format string=w1146:string[])  [unwired: 2 in]
            n439 = case shown="False" w1161 {
              tunnel: w1162 -> [w1181 w1200]
              tunnel: w1150 -> [w1182 w1199]
              tunnel: [w1184 w1198] -> w1159
              tunnel: [w1183 w1197] -> w1157
              tunnel: w1160 -> [w1180 _]
              tunnel: w1146 -> [w1176 w1189]
              tunnel: w1145 -> [w1172 w1188]
              frame False {
                # "DO TRACEBILITY"
                n440 = Index Array(array=w1172) -> (element #1=w1173:string, element #2=w1170:string, element #3=w1168:string)  [unwired: 3 in]
                n441 = call <vilib>:"Trim Whitespace.vi"("string"=w1173) -> ("trimmed string"=w1174:string)  [unwired: 1 in]
                n442 = local read "SHIFT"() -> (w1167:string)
                n443 = Index Array(array=w1176) -> (element #1=w1171:string, element #2=w1169:string)  [unwired: 2 in]
                n444 = call "PADMINI_SHIFT_DATE.vi"("SHIFT"=w1167) -> ("date/time string"=w1166:string)  [unwired: 10 in]
                n445 = Bundle("date/time string"=w1166, "Input 2"=w1171, "Input 2"=w1170, "Input 2"=w1169, "Input 2"=w1168) -> (w1175:T19)  [unwired: 1 in]
                n446 = Format Into String(format string="Where BARCODE='%s' ", w1174) -> (resulting string=w1178:string)  [unwired: 2 in, 1 out]
                n447 = call <vilib>:"DB Tools Update Data.vi"("condition"=w1178, "data"=w1175, "error in (no error)"=w1182, "columns"=string[] ["DATE_OP90", "OP90_SEAT_LEAK", "OP90_SEAT_STATUS", "OP90_STEAM_LEAK", "OP90_FINAL_RST"], "table"=w1180, "connection reference"=w1181) -> ("error out"=w1183:errorcluster, "connection reference out"=w1184:T13)  [unwired: 4 in]
              }
              frame True {
                # "TRAC BYPASS"
                n448 = local read "SHIFT"() -> (w1185:string)
                n449 = call "PADMINI_SHIFT_DATE.vi"("SHIFT"=w1185) -> ("date/time string"=w1186:string)  [unwired: 10 in]
                n450 = Index Array(array=w1188) -> (element #2=w1193:string, element #3=w1191:string)  [unwired: 3 in, 1 out]
                n451 = Index Array(array=w1189) -> (element #1=w1194:string, element #2=w1192:string)  [unwired: 2 in]
                n452 = Bundle("date/time string"=w1186, "SHIFT"=w1185, "Input 2"=w1194, "Input 2"=w1193, "Input 2"=w1192, "Input 2"=w1191) -> (w1190:T20)  [unwired: 1 in]
                n453 = To Variant(anything=w1190) -> (Variant=w1196:variant)
                n454 = call <vilib>:"DB Tools Insert Data.vi"("data"=w1196, "error in (no error)"=w1199, "columns"=string[] ["DATE", "SHIFT", "ST9_SEAT_LT_DATA", "ST9_SEAT_STATUS", "ST9_STEAM_LT_DATA", "ST9_FINAL_RST"], "table"="ST9_REPORT", "connection reference"=w1200) -> ("error out"=w1197:errorcluster, "connection reference out"=w1198:T13)  [unwired: 5 in]
              }
            }
            n455 = call <vilib>:"Simple Error Handler.vi"("type of dialog (OK msg:1)"=w1156, "error in (no error)"=w1157) -> ("error out"=w1155:errorcluster)  [unwired: 3 in, 4 out]
            n456 = call <vilib>:"Clear Errors.vi"("error in (no error)"=w1155) -> ("error out"=w1153:errorcluster)  [unwired: 5 in, 1 out]
            n457 = flat-sequence {
              tunnel: [w1165] -> w1143
              tunnel: w1153 -> [w1165]
              frame #0 {
                # "UPDATE op 20 save"
                n458 = global write "DATA LOG.vi" "OP 90 reset"(TRUE) -> ()
              }
            }
          }
          frame "SCAN10" {
            # "STATION OP 10"
            n459 = case shown="False" w1207 {
              tunnel: w1211 -> [w1230 w1236]
              tunnel: w1210 -> [w1224 w1235]
              tunnel: w1209 -> [w1216 _]
              tunnel: [w1213 w1234] -> w1206
              tunnel: [w1225 w1236] -> w1208
              tunnel: [w1217 "" ("trimmed string")] -> _
              frame False {
                (unwired) "REPORT"
                n460 = call "PADMINI_AUTO_BARCODE_STRING 100.vi"("Enum"=enum16{"Read", "Write"}."Read", "error in (no error)"=w1224) -> ("error out"=w1223:errorcluster, "Input 2"=w1219:string[])  [unwired: 8 in]
                n461 = Index Array(array=w1219) -> (element=w1218:string)  [unwired: 1 in]
                n462 = call <vilib>:"Trim Whitespace.vi"("string"=w1218) -> ("trimmed string"=w1217:string)  [unwired: 1 in]
                n463 = Format Into String(format string="WHERE BARCODE  ='%s'", w1217) -> (resulting string=w1220:string)  [unwired: 2 in, 1 out]
                n464 = call <vilib>:"DB Tools Select Data.vi"("condition"=w1220, "error in (no error)"=w1223, "columns"=string[] ["BARCODE", "OP90_FINAL_RST", "OP100_FINAL_RST"], "table"=w1216, "connection reference"=w1230) -> ("error out"=w1228:errorcluster, "data"=w1227:variant[][], "connection reference out"=w1225:T13)  [unwired: 1 in]
                n465 = call "PADMINI_varient_to_data.vi"("error in (no error)"=w1228, "data"=w1227) -> ("error out"=w1226:errorcluster, "Array"=w1215:string[][])  [unwired: 8 in]
                n466 = call "RESPONSE_LOGIC.vi"("Array"=w1215) -> ("Not Found"=w1212:i32[])  [unwired: 10 in]
                n467 = call "PADMINI_AUTO_BARCODE_STATUS 100.vi"("Enum"=enum16{"Read", "Write"}."Write", "error in (no error)"=w1226, "I/P"=w1212) -> ("error out"=w1213:errorcluster)  [unwired: 7 in, 1 out]
              }
              frame True {
                w1231 = i32[] [0, 0, 0, 0, 0]  # I/P
                n468 = call "PADMINI_AUTO_BARCODE_STATUS 100.vi"("Enum"=enum16{"Read", "Write"}."Write", "error in (no error)"=w1235, "I/P"=w1231) -> ("error out"=w1234:errorcluster)  [unwired: 7 in, 1 out]
              }
            }
            n469 = flat-sequence {
              tunnel: [w1238] -> w1205
              tunnel: w1206 -> [w1238]
              frame #0 {
                # "UPDATE op 100 SCAN sTATUS"
                n470 = global write "DATA LOG.vi" "OP 100 Outputs"(TRUE) -> ()
              }
            }
          }
          frame "SCAN11" {
            # "STATION OP 110"
            n471 = case shown="False" w1245 {
              tunnel: w1249 -> [w1276 w1286]
              tunnel: w1248 -> [w1269 w1285]
              tunnel: w1247 -> [w1261 _]
              tunnel: [w1271 w1284] -> w1244
              tunnel: [w1270 w1286] -> w1246
              frame False {
                w1254 = 0  # disabled index (col)
                (unwired) "REPORT"
                # "OP100 OK\nOP 100 NG"
                n472 = call "PADMINI_AUTO_BARCODE_STRING 100.vi"("Enum"=enum16{"Read", "Write"}."Read", "error in (no error)"=w1269) -> ("error out"=w1268:errorcluster, "Input 2"=w1263:string[])  [unwired: 8 in]
                n473 = Index Array(array=w1263) -> (element=w1262:string)  [unwired: 1 in]
                n474 = call <vilib>:"Trim Whitespace.vi"("string"=w1262) -> ("trimmed string"=w1264:string)  [unwired: 1 in]
                n475 = Format Into String(format string="WHERE BARCODE  ='%s'", w1264) -> (resulting string=w1265:string)  [unwired: 2 in, 1 out]
                n476 = call <vilib>:"DB Tools Select Data.vi"("condition"=w1265, "error in (no error)"=w1268, "columns"=string[] ["BARCODE", "OP100_FINAL_RST"], "table"=w1261, "connection reference"=w1276) -> ("error out"=w1274:errorcluster, "data"=w1273:variant[][], "connection reference out"=w1270:T13)  [unwired: 1 in]
                n477 = call "PADMINI_varient_to_data.vi"("error in (no error)"=w1274, "data"=w1273) -> ("error out"=w1272:errorcluster, "Array"=w1250:string[][])  [unwired: 8 in]
                n478 = Index Array(array=w1250, index (row)=w1254) -> (element=w1255:string[])  [unwired: 1 in]
                n479 = Index Array(array=w1255) -> (element #1=w1259:string, element #2=w1256:string)  [unwired: 2 in]
                n480 = Equal?(x="", y=w1259) -> (x = y?=w1258:bool)
                n481 = Equal?(x=w1256, y="OK") -> (x = y?=w1257:bool)
                n482 = case shown="True" w1258 {
                  tunnel: w1257 -> [w1277 _]
                  tunnel: [w1278 w1281] -> w1251
                  frame False {
                    # "BARCODE FOUND"
                    n483 = case shown="False" w1277 {
                      tunnel: [w1279 w1280] -> w1278
                      frame False {
                        w1279 = i32[] [0, 1]  # OK
                        # "CT ST REPEAT NG & EMPTY"
                      }
                      frame True {
                        w1280 = i32[] [1, 0]  # NG
                        # "CT ST REPEAT EMPTY"
                      }
                    }
                  }
                  frame True {
                    w1281 = i32[] [0, 1]  # Not Found
                    # "nO BARCODE FOUND"
                  }
                }
                n484 = call "PADMINI_AUTO_BARCODE_STATUS 110.vi"("Enum"=enum16{"Read", "Write"}."Write", "error in (no error)"=w1272, "I/P"=w1251) -> ("error out"=w1271:errorcluster)  [unwired: 7 in, 1 out]
              }
              frame True {
                w1282 = i32[] [0, 0, 0, 0, 0]  # I/P
                n485 = call "PADMINI_AUTO_BARCODE_STATUS 100.vi"("Enum"=enum16{"Read", "Write"}."Write", "error in (no error)"=w1285, "I/P"=w1282) -> ("error out"=w1284:errorcluster)  [unwired: 7 in, 1 out]
              }
            }
            n486 = flat-sequence {
              tunnel: [w1288] -> w1243
              tunnel: w1244 -> [w1288]
              frame #0 {
                # "UPDATE op 100 SCAN sTATUS"
                n487 = global write "DATA LOG.vi" "OP 110 Outputs"(TRUE) -> ()
              }
            }
          }
          frame "DATALOG10" {
            w1302 = T14 2 items=["no dialog", "OK message", "continue or stop message", "OK message + warnings", "continue/stop + warnings"] ("type of dialog (OK msg:1)")
            # "datalog of OP 100"
            n488 = call "PADMINI_AUTO_BARCODE_STRING 100.vi"("Enum"=enum16{"Read", "Write"}."Read", "error in (no error)"=w1290) -> ("error out"=w1296:errorcluster, "Input 2"=w1292:string[])  [unwired: 8 in]
            n489 = call "PADMINI_AUTO_CYCLE VALUE 100.vi"("Enum"=enum16{"Read", "Write"}."Read", "error in (no error)"=w1290) -> ("Input 2"=w1291:sgl[])  [unwired: 8 in, 1 out]
            n490 = Number To Fractional String(number=w1291, precision (6)=i16 2) -> (F-format string=w1293:string[])  [unwired: 2 in]
            n491 = case shown="False" w1307 {
              tunnel: w1308 -> [w1335 w1360]
              tunnel: w1296 -> [w1336 w1359]
              tunnel: [w1338 w1358] -> w1305
              tunnel: [w1337 w1357] -> w1303
              tunnel: w1306 -> [w1334 _]
              tunnel: w1293 -> [w1330 w1342]
              tunnel: w1292 -> [w1327 w1343]
              frame False {
                # "DO TRACEBILITY"
                n492 = Index Array(array=w1327) -> (element #1=w1326:string, element #2=w1312:string)  [unwired: 2 in]
                n493 = call <vilib>:"Trim Whitespace.vi"("string"=w1326) -> ("trimmed string"=w1328:string)  [unwired: 1 in]
                n494 = Index Array(array=w1330) -> (element #1=w1323:string, element #2=w1322:string, element #3=w1321:string, element #4=w1320:string, element #5=w1319:string, element #6=w1318:string, element #7=w1317:string, element #8=w1316:string, element #9=w1315:string, element #10=w1314:string, element #11=w1313:string)  [unwired: 11 in]
                n495 = local read "SHIFT"() -> (w1325:string)
                n496 = call "PADMINI_SHIFT_DATE.vi"("SHIFT"=w1325) -> ("date/time string"=w1324:string)  [unwired: 10 in]
                n497 = Bundle("date/time string"=w1324, "Input 2"=w1323, "Input 2"=w1322, "Input 2"=w1321, "Input 2"=w1320, "Input 2"=w1319, "Input 2"=w1318, "Input 2"=w1317, "Input 2"=w1316, "Input 2"=w1315, "Input 2"=w1314, "Input 2"=w1313, "Input 2"=w1312) -> (w1329:T25)  [unwired: 1 in]
                n498 = Format Into String(format string="Where BARCODE='%s' ", w1328) -> (resulting string=w1332:string)  [unwired: 2 in, 1 out]
                n499 = call <vilib>:"DB Tools Update Data.vi"("condition"=w1332, "data"=w1329, "error in (no error)"=w1336, "columns"=string[] ["DATE_OP100", "OP100_SENSOR_OP_OPEN", "OP100_SENSOR_OP_CLOSE", "OP100_SENSOR_OP_FULL_CLOSE", "OP100_SENSOR_INITIAL", "OP100_MOTOR_START_OF_CLOSE", "OP100_MOTOR_FULL_CLOSE", "OP100_MOTOR_START_BACK", "OP100_MOTOR_FULL_OPEN", "OP100_RESPONSE_TIME_FWD", "OP100_RESPONSE_TIME_REV", "OP100_MOTOR_PEAK_CURRENT", "OP100_FINAL_RST"], "table"=w1334, "connection reference"=w1335) -> ("error out"=w1337:errorcluster, "connection reference out"=w1338:T13)  [unwired: 4 in]
              }
              frame True {
                # "TRAC BYPASS"
                n500 = local read "SHIFT"() -> (w1340:string)
                n501 = Index Array(array=w1343) -> (element=w1347:string)  [unwired: 1 in]
                n502 = call "PADMINI_SHIFT_DATE.vi"("SHIFT"=w1340) -> ("date/time string"=w1341:string)  [unwired: 10 in]
                n503 = Index Array(array=w1342) -> (element #1=w1353:string, element #2=w1352:string, element #3=w1339:string, element #4=w1345:string, element #5=w1351:string, element #6=w1346:string, element #7=w1350:string, element #8=w1349:string, element #9=w1348:string)  [unwired: 9 in]
                n504 = Bundle("date/time string"=w1341, "SHIFT"=w1340, "Input 2"=w1353, "Input 2"=w1352, "Input 2"=w1339, "Input 2"=w1339, "Input 2"=w1339, "Input 2"=w1345, "Input 2"=w1351, "Input 2"=w1346, "Input 2"=w1350, "Input 2"=w1349, "Input 2"=w1348, "Input 2"=w1347) -> (w1344:T26)  [unwired: 1 in]
                n505 = To Variant(anything=w1344) -> (Variant=w1356:variant)
                n506 = call <vilib>:"DB Tools Insert Data.vi"("data"=w1356, "error in (no error)"=w1359, "columns"=string[] ["DATE", "SHIFT", "ST10_SENSOR_OP_OPEN_V", "ST10_START_OF_CLOSE_SENSOR_V", "ST10_SENSOR_OP_FULL_CLOSE_V", "ST10_RESPONSE_TIME_FWD", "ST10_RESPONSE_TIME_REV", "ST10_MOTOR_V_START_OF_CLOSE_A", "ST10_MOTOR_V_FULL_CLOSE_B", "ST10_MOTOR_V_START_BACK_C", "ST10_MOTOR_V_FULL_OPEN_D", "ST10_MOTOR_RMS_CURRENT_A", "ST10_FINAL_RST"], "table"="ST10_REPORT", "connection reference"=w1360) -> ("error out"=w1357:errorcluster, "connection reference out"=w1358:T13)  [unwired: 5 in]
              }
            }
            n507 = call <vilib>:"Simple Error Handler.vi"("type of dialog (OK msg:1)"=w1302, "error in (no error)"=w1303) -> ("error out"=w1301:errorcluster)  [unwired: 3 in, 4 out]
            n508 = call <vilib>:"Clear Errors.vi"("error in (no error)"=w1301) -> ("error out"=w1299:errorcluster)  [unwired: 5 in, 1 out]
            n509 = flat-sequence {
              tunnel: [w1311] -> w1289
              tunnel: w1299 -> [w1311]
              frame #0 {
                # "UPDATE op 20 save"
                n510 = global write "DATA LOG.vi" "OP 100 reset"(TRUE) -> ()
              }
            }
          }
          frame "EMERGENCY STOP" {
          }
          frame "STOP" {
            n511 = global read "Global 1.vi" "BARCODE RECIPE"() -> (w1371:string)
            n512 = Bundle("BARCODE RECIPE"=w1371) -> (w1370:cluster{"BARCODE RECIPE":string})  [unwired: 1 in]
            n513 = call <vilib>:"DB Tools Update Data.vi"("data"=w1370, "error in (no error)"=w1376, "columns"=string[] ["PREVIOUS_LOADED_RECIPE"], "table"="BARCODE_RECIPE", "connection reference"=w1374) -> ("error out"=w1375:errorcluster, "connection reference out"=w1373:T13)  [unwired: 5 in]
          }
        }
      }
      frame Error {
        # "Return true in any case that should stop the loop."
      }
    }
    n514 = Unbundle By Name(w130) -> ("OP - 90"=→"OP - 90":T29, "OP - 100"=→"OP - 100":T30, "OP - 110"=→"OP - 110":cluster{"BARCODE":string})
    n515 = Unbundle By Name(w130) -> ("OP - 10"=→"OP - 10":T31, "OP - 20"=→"OP - 20":T5, "OP - 30"=→"OP - 30":T32, "OP - 40"=→"OP - 40":T2)
    n516 = Unbundle By Name(w130) -> ("OP - 50"=→"OP - 50":T1, "OP - 60"=→"OP - 60":T33, "OP - 70"=→"OP - 70":T34, "OP - 80"=→"OP - 80":T35)
    n517 = Wait (ms)(milliseconds to wait=u32 100) -> ()  [unwired: 1 out]
    n518 = call <vilib>:"Simple Error Handler.vi"("error in (no error)"=w124) -> ("error out"=w123:errorcluster)  [unwired: 4 in, 4 out]
  }
  n519 = while {
    shift-right: [w1400] -> w72
    shift-left: w22 -> [w1394]
    shift-right: [w1401] -> w66
    shift-left: w70 -> [w1409]
    stop <- w1399 stop-if-true
    n520 = local read "Shift_change"() -> (w1407:bool)
    n521 = call <vilib>:"Clear Errors.vi"("error in (no error)"=w1394) -> ("error out"=w1385:errorcluster)  [unwired: 5 in, 1 out]
    n522 = call "READ EMERGENCY BIT.vi"("Enum"=enum16{"Read", "Write"}."Read", "error in (no error)"=w1385) -> ("Array Out"=w1397:dbl[])  [unwired: 8 in, 1 out]
    n523 = case shown="True" w1407 {
      tunnel: w1385 -> [w1426 w1439]
      tunnel: [w1427 w1438] -> w1406
      frame False {
        n524 = local read "SHIFT_DATA 2"() -> (w1429:string[])
        n525 = Get Date/Time In Seconds() -> (seconds since 1Jan1904=w1428:timestamp)
        n526 = call "String To Time_4.vi"("error in (no error)"=w1426, "String Array In"=w1429) -> ("error out"=w1425:errorcluster, "Time Stamp Out"=w1424:timestamp[])  [unwired: 8 in]
        "Time Stamp Out 4" <- w1424
        n527 = call "Shift Calculation_4.vi"("error in (no error)"=w1425, "Current Time"=w1428, "Time Stamp Out"=w1424) -> ("error out"=w1423:errorcluster, "Shift"=w1422:i32)  [unwired: 7 in]
        n528 = call <vilib>:"Clear Errors.vi"("error in (no error)"=w1423) -> ()  [unwired: 5 in, 2 out]
        n529 = case shown="4" w1422 {
          tunnel: ["A" "B" "C" "D"] -> w1427
          frame 1, Default {
          }
          frame 2 {
          }
          frame 3 {
          }
          frame 4 {
          }
        }
      }
      frame True {
        n530 = local read "SHIFT_DATA"() -> (w1437:string[])
        n531 = Get Date/Time In Seconds() -> (seconds since 1Jan1904=w1440:timestamp)
        n532 = call "String To Time.vi"("error in (no error)"=w1439, "String Array In"=w1437) -> ("error out"=w1436:errorcluster, "Time Stamp Out"=w1441:timestamp[])  [unwired: 8 in]
        "Time Stamp Out" <- w1441
        n533 = call "Shift Calculation.vi"("error in (no error)"=w1436, "Current Time"=w1440, "Time Stamp Out"=w1441) -> ("error out"=w1435:errorcluster, "Shift"=w1434:i32)  [unwired: 7 in]
        "Shift 4" <- w1434
        n534 = call <vilib>:"Clear Errors.vi"("error in (no error)"=w1435) -> ()  [unwired: 5 in, 2 out]
        n535 = case shown="3" w1434 {
          tunnel: ["A" "B" "C"] -> w1438
          frame 1, Default {
          }
          frame 2 {
          }
          frame 3 {
          }
        }
      }
    }
    "SHIFT" <- w1406
    n536 = Index Array(array=w1397) -> (element=w1396:dbl)  [unwired: 1 in]
    n537 = call "VALUE_CHANGE - ST1_RESULT.vi"("Numeric"=w1396) -> ("Boolean"=w1395:bool)  [unwired: 9 in, 1 out]
    n538 = global write "Global 1.vi" "EMERGENCY STOP"(w1395) -> ()
    n539 = call "Trigger_Loggic.vi"("error in (no error)"=w1385) -> ("error out"=w1390:errorcluster, "Array"=w1410:i32[])  [unwired: 9 in]
    n540 = for {
      tunnel: w1410 -> [w1445] mode=indexing
      shift-right: [w1449] -> w1403
      shift-left: w1409 -> [w1448]
      shift-right: [w1447] -> w1402
      shift-left: w1390 -> [w1446]
      n541 = case shown="0" w1445 {
        tunnel: [w1452 w1457 w1461 w1467 w1472 w1477 w1482 w1487 w1492 w1497 w1502 w1507 w1512 w1517 w1522 w1527 w1532 w1537 w1542 w1547 w1552 w1557 w1562] -> w1449
        tunnel: w1448 -> [w1454 w1459 w1462 w1469 w1474 w1479 w1484 w1489 w1494 w1499 w1504 w1509 w1514 w1519 w1524 w1529 w1534 w1539 w1544 w1549 w1554 w1559 w1564]
        tunnel: [w1451 w1456 w1463 w1466 w1471 w1476 w1481 w1486 w1491 w1496 w1501 w1506 w1511 w1516 w1521 w1526 w1531 w1536 w1541 w1546 w1551 w1556 w1561] -> w1447
        tunnel: w1446 -> [w1453 w1458 w1464 w1468 w1473 w1478 w1483 w1488 w1493 w1498 w1503 w1508 w1513 w1518 w1523 w1528 w1533 w1538 w1543 w1548 w1553 w1558 w1563]
        frame -1, Default {
          # "DEFAULT"
          n542 = Enqueue Element(queue=w1454, element=cluster{"CASE 2":T12} {"CASE 2"=enum."-1"}, error in (no error)=w1453) -> (queue out=w1452:refnum<queue>, error out=w1451:errorcluster)  [unwired: 1 in, 1 out]
        }
        frame 0 {
          # "SCAN BARCODE OP 10"
          n543 = Enqueue Element(queue=w1459, element=cluster{"CASE 2":T12} {"CASE 2"=enum."-1"}, error in (no error)=w1458) -> (queue out=w1457:refnum<queue>, error out=w1456:errorcluster)  [unwired: 1 in, 1 out]
        }
        frame 1 {
          # "DATALOG OF OP 10"
          n544 = Enqueue Element(queue=w1462, element=cluster{"CASE 2":T12} {"CASE 2"=enum."SCAN1"}, error in (no error)=w1464) -> (queue out=w1461:refnum<queue>, error out=w1463:errorcluster)  [unwired: 1 in, 1 out]
        }
        frame 2 {
          # "SCAN BARCODE OP 20"
          n545 = Enqueue Element(queue=w1469, element=cluster{"CASE 2":T12} {"CASE 2"=enum."SCAN2"}, error in (no error)=w1468) -> (queue out=w1467:refnum<queue>, error out=w1466:errorcluster)  [unwired: 1 in, 1 out]
        }
        frame 3 {
          # "DATALOG OF OP 20"
          n546 = Enqueue Element(queue=w1474, element=cluster{"CASE 2":T12} {"CASE 2"=enum."DATALOG2"}, error in (no error)=w1473) -> (queue out=w1472:refnum<queue>, error out=w1471:errorcluster)  [unwired: 1 in, 1 out]
        }
        frame 4 {
          # "SCAN BARCODE OP 30"
          n547 = Enqueue Element(queue=w1479, element=cluster{"CASE 2":T12} {"CASE 2"=enum."SCAN3"}, error in (no error)=w1478) -> (queue out=w1477:refnum<queue>, error out=w1476:errorcluster)  [unwired: 1 in, 1 out]
        }
        frame 5 {
          # "DATALOG OF OP 30"
          n548 = Enqueue Element(queue=w1484, element=cluster{"CASE 2":T12} {"CASE 2"=enum."DATALOG3"}, error in (no error)=w1483) -> (queue out=w1482:refnum<queue>, error out=w1481:errorcluster)  [unwired: 1 in, 1 out]
        }
        frame 6 {
          # "SCAN BARCODE OP 40"
          n549 = Enqueue Element(queue=w1489, element=cluster{"CASE 2":T12} {"CASE 2"=enum."SCAN4"}, error in (no error)=w1488) -> (queue out=w1487:refnum<queue>, error out=w1486:errorcluster)  [unwired: 1 in, 1 out]
        }
        frame 7 {
          # "DATALOG OF OP 40"
          n550 = Enqueue Element(queue=w1494, element=cluster{"CASE 2":T12} {"CASE 2"=enum."DATALOG4"}, error in (no error)=w1493) -> (queue out=w1492:refnum<queue>, error out=w1491:errorcluster)  [unwired: 1 in, 1 out]
        }
        frame 8 {
          # "SCAN BARCODE OP 50"
          n551 = Enqueue Element(queue=w1499, element=cluster{"CASE":T12} {"CASE"=enum."SCAN5"}, error in (no error)=w1498) -> (queue out=w1497:refnum<queue>, error out=w1496:errorcluster)  [unwired: 1 in, 1 out]
        }
        frame 9 {
          # "DATALOG OF OP 50"
          n552 = Enqueue Element(queue=w1504, element=cluster{"CASE":T12} {"CASE"=enum."DATALOG5"}, error in (no error)=w1503) -> (queue out=w1502:refnum<queue>, error out=w1501:errorcluster)  [unwired: 1 in, 1 out]
        }
        frame 10 {
          # "SCAN BARCODE OP 60"
          n553 = Enqueue Element(queue=w1509, element=cluster{"CASE 2":T12} {"CASE 2"=enum."SCAN6"}, error in (no error)=w1508) -> (queue out=w1507:refnum<queue>, error out=w1506:errorcluster)  [unwired: 1 in, 1 out]
        }
        frame 11 {
          # "DATALOG OF OP 60"
          n554 = Enqueue Element(queue=w1514, element=cluster{"CASE 2":T12} {"CASE 2"=enum."DATALOG6"}, error in (no error)=w1513) -> (queue out=w1512:refnum<queue>, error out=w1511:errorcluster)  [unwired: 1 in, 1 out]
        }
        frame 12 {
          # "SCAN BARCODE OP 70"
          n555 = Enqueue Element(queue=w1519, element=cluster{"CASE 2":T12} {"CASE 2"=enum."SCAN7"}, error in (no error)=w1518) -> (queue out=w1517:refnum<queue>, error out=w1516:errorcluster)  [unwired: 1 in, 1 out]
        }
        frame 13 {
          # "DATALOG OF OP 70"
          n556 = Enqueue Element(queue=w1524, element=cluster{"CASE 2":T12} {"CASE 2"=enum."DATALOG7"}, error in (no error)=w1523) -> (queue out=w1522:refnum<queue>, error out=w1521:errorcluster)  [unwired: 1 in, 1 out]
        }
        frame 14 {
          # "SCAN BARCODE 80"
          n557 = Enqueue Element(queue=w1529, element=cluster{"CASE 2":T12} {"CASE 2"=enum."SCAN8"}, error in (no error)=w1528) -> (queue out=w1527:refnum<queue>, error out=w1526:errorcluster)  [unwired: 1 in, 1 out]
        }
        frame 15 {
          # "DATALOG OF OP 80"
          n558 = Enqueue Element(queue=w1534, element=cluster{"CASE 2":T12} {"CASE 2"=enum."DATALOG8"}, error in (no error)=w1533) -> (queue out=w1532:refnum<queue>, error out=w1531:errorcluster)  [unwired: 1 in, 1 out]
        }
        frame 16 {
          # "SCAN BARCODE OP 90"
          n559 = Enqueue Element(queue=w1539, element=cluster{"CASE 2":T12} {"CASE 2"=enum."SCAN9"}, error in (no error)=w1538) -> (queue out=w1537:refnum<queue>, error out=w1536:errorcluster)  [unwired: 1 in, 1 out]
        }
        frame 17 {
          # "DATALOG OF OP 90"
          n560 = Enqueue Element(queue=w1544, element=cluster{"CASE 2":T12} {"CASE 2"=enum."DATALOG9"}, error in (no error)=w1543) -> (queue out=w1542:refnum<queue>, error out=w1541:errorcluster)  [unwired: 1 in, 1 out]
        }
        frame 18 {
          # "SCAN BARCODE OP 100"
          n561 = Enqueue Element(queue=w1549, element=cluster{"CASE 2":T12} {"CASE 2"=enum."SCAN10"}, error in (no error)=w1548) -> (queue out=w1547:refnum<queue>, error out=w1546:errorcluster)  [unwired: 1 in, 1 out]
        }
        frame 19 {
          # "DATALOG OF OP 100"
          n562 = Enqueue Element(queue=w1554, element=cluster{"CASE 2":T12} {"CASE 2"=enum."DATALOG10"}, error in (no error)=w1553) -> (queue out=w1552:refnum<queue>, error out=w1551:errorcluster)  [unwired: 1 in, 1 out]
        }
        frame 20 {
          # "SCAN BARCODE OP 110"
          n563 = Enqueue Element(queue=w1559, element=cluster{"CASE 2":T12} {"CASE 2"=enum."SCAN11"}, error in (no error)=w1558) -> (queue out=w1557:refnum<queue>, error out=w1556:errorcluster)  [unwired: 1 in, 1 out]
        }
        frame 21 {
          # "DATALOG OF OP 110"
          n564 = Enqueue Element(queue=w1564, element=cluster{"CASE 2":T12} {"CASE 2"=enum."DATALOG11"}, error in (no error)=w1563) -> (queue out=w1562:refnum<queue>, error out=w1561:errorcluster)  [unwired: 1 in, 1 out]
        }
      }
    }
    n565 = Wait (ms)(milliseconds to wait=u32 50) -> ()  [unwired: 1 out]
    n566 = global read "Global 1.vi" "PLC COMM"() -> (→"PLC COM.":bool)
    n567 = global read "Global 1.vi" "PLC 1"() -> (→"OP 10 & 20":bool)
    n568 = global read "Global 1.vi" "PLC 2"() -> (→"OP 30":bool)
    n569 = global read "Global 1.vi" "PLC 3"() -> (→"OP 40":bool)
    n570 = case shown="False" "stop 2" {
      tunnel: w1403 -> [w1413 w1419]
      tunnel: [w1413 w1418] -> w1401
      tunnel: w1402 -> [w1412 w1417]
      tunnel: [w1412 w1416] -> w1400
      tunnel: [FALSE TRUE] -> w1399
      frame False {
      }
      frame True {
        n571 = Flush Queue(queue=w1419, error in (no error)=w1417) -> (queue out=w1421:refnum<queue>, error out=w1420:errorcluster)  [unwired: 1 out]
        n572 = Enqueue Element(queue=w1421, element=cluster{"CASE 2":T12} {"CASE 2"=enum."STOP"}, error in (no error)=w1420) -> (queue out=w1418:refnum<queue>, error out=w1416:errorcluster)  [unwired: 1 in, 1 out]
      }
    }
    "stop" <- w1399
    n573 = global read "Global 1.vi" "PLC 4"() -> (→"OP 50":bool)
    n574 = global read "Global 1.vi" "PLC 5"() -> (→"OP 60":bool)
    n575 = global read "Global 1.vi" "PLC 7"() -> (→"OP 90 -100 - 110":bool)
    n576 = global read "Global 1.vi" "PLC 6"() -> (→"OP 70 & 80":bool)
  }
  n577 = Release Queue(queue=w66, error in (no error)=w72) -> (error out=w49:errorcluster)  [unwired: 1 in, 2 out]
  n578 = call <vilib>:"Clear Errors.vi"("error in (no error)"=w68) -> ("error out"=w53:errorcluster)  [unwired: 5 in, 1 out]
  n579 = call <vilib>:"DB Tools Close Connection.vi"("error in (no error)"=w53, "connection reference"=w67) -> ("error out"=w50:errorcluster)  [unwired: 5 in]
  n580 = Merge Errors(w49, w50) -> (w51:errorcluster)
  n581 = call <vilib>:"Simple Error Handler.vi"("error in (no error)"=w51) -> ("error out"=w46:errorcluster)  [unwired: 4 in, 4 out]
  n582 = call <vilib>:"Clear Errors.vi"("error in (no error)"=w46) -> ("error out"=w52:errorcluster)  [unwired: 5 in, 1 out]
  n583 = flat-sequence {
    tunnel: w52 -> [w1567]
    tunnel: [w1567] -> w54
    frame #0 {
      n584 = global write "Global 1.vi" "REMOVE VI"(TRUE ("remove_VI")) -> ()
      n585 = global write "DATA LOG.vi" "Auto Cycle On"(FALSE) -> ()
    }
  }
  n586 = property class="App"(error in=w54) -> (error out=w56:errorcluster, "App.Kind"=w55:T36)  [unwired: 1 in, 1 out]
  n587 = case shown="\"Run Time System\"" w55 {
    tunnel: [w1568 w1570] -> w57
    tunnel: w56 -> [w1568 w1569]
    frame "Development System", Default {
    }
    frame "Run Time System" {
      n588 = invoke class="VI" method="FP.Close"(error in=w1569) -> (error out=w1570:errorcluster)  [unwired: 2 in, 2 out]
    }
  }
  "error out 2" <- w57
